vi "Argos_K_0v8.vi"(0 "PID 1 COM":refnum<visa-resource-name>="COM1", 1 "Setpoint\n START":bool, 2 "Write to File":bool, 3 "SP 1 input (°C)":dbl=20.0 min=0.0 max=1300.0, 4 "Intervall (s)":u32=1 max=600, 5 "Write/\nRead":bool=TRUE, 6 "Delay (ms)":u32=500 min=100 max=600000, 7 "Auto Tune":bool, 9 "Standby":bool, 11 "Reset\nSTOP":bool, 12 "ON":bool=TRUE caption="OFF", 13 "Get Values":bool, 15 "File Path":path) -> (8 "(°C)":dbl format="%#.3f", 14 "SP 1 is (°C)":dbl)   [LabVIEW 2013]
doc: "1. Verwendung\n\nDas Programm dient der Steuerung und Abfrage des Thermocontrollers I3252 und dem Auslesen von zwei VC 840 Messgeräten und einem Druckmessgerät Pfeiffer Single Gauge. \nDie Messgeräte werden Standardmäßig ausgelesen und erst nach Betätigung des Schalters \"Write to File\" in einer Textdatei abgespeichert. Das Eingabefeld \"Intervall\" legt den Abstand der Messpunkte fest.\nDer Setpoint für den Thermocontroller wird erst nach Betätigung des Tasters \"Setpoint START\" übernommen und angesteuert. Er wird ind den EEPROM des Gerätes geschrieben. Die Regelung kann mit Hilfe des Schalters \"Standby\" unterbrochen werden. Durch den Taster \"Reset STOPP\" kann der Setpoint aus dem EEPROM gelöscht werden.\nDie Eingabeflächen \"Constant\" und \"Thickness\" dienen der Berechnung des spezifischen Widerstands.\nDie Eingabeflächen \"User\" und \"Sample\" werden in den Header der Textdatei übernommen.\nDer Indikator \"File Path\" zeigt den aktuellen Speicherort der Textdatei an. Dieser wird nach ausschalten des Schalters \"Write to File\" gelöscht. Bei erneuten Schreiben muss ein neuer Speicherort gewählt werden. Bei Wahl desselben Speicherorts werden sämtliche bereits gespeicherte Daten gelöscht.\n\n\n2. Erläuterungen zum Blockdiagramm\n2.1 äußere Sequenz\nDie äußerte Sequenz besteht aus fünf Frames. Der erste dient der Initialisierung der Ports. Der zweite dient als Verzögerung um dem Programm genug Zeit zu geben die Ports zu öffnen. Jedoch senden die beiden VC 840 bereits Informationen an den Computer die in einem Puffer zwischengespeichert werden. Im dritten Frame wird dieser Puffer geleert. Somit kommt es zu keinem Framing Error. Desweiteren wird in diesem Frame die Startzeit der Messungen genommen. Im vierten Frame wird die eigentliche Messung und Verarbeitung der Daten durchgeführt. Die while-Schleife wird nur durch Auftreten eines Fehlers oder durch Betätigung des Stopbuttons auf dem Front Panel in der oberen linken Ecke unterbrochen. Im fünften und letzten Frame werden die Ports wieder geschlossen und beim Auftreten eines Fehlers wird das Programm automatisch gestoppt. Falls kein Fehler auftritt wird die Sequenz von vorne abgearbeitet.\n\n2.2 while-Schleife und innere Sequenz\n2.2.1 \"Event Structure\"\n2.2.1.1 Allgemein\nDer erste Frame beinhaltet ein \"Event Structure\". Dieser reagiert auf insgesamt elf verschiedene Ereignisse. Falls keines dieser Ereignisse auftreten sollte, warte die Struktur eine Millisekunde bevor die \"Event Structure\" verlassen wird. Die übrigen Ereignisse treten ein, wenn der entsprechende Kontroller eine Werteänderung erfährt.\n\n2.2.1.2 Event: Setpoint\nDieser Case besteht von außen nach innen aus einer Stacked Sequence, einer for-Loop und einer Flat Sequence die wiederum zwei \"Case Structures\" enthält. Als erstes wird bei dem Schalter \"Setpoint START\" der Blinkmodus aktiviert und bei dem Schalter \"Read Temperature\" deaktiviert. Danach folgt das eigentliche setzen des Temperatursollwerts. In der ersten Iteration wird dem Controller I3252 ein Schreibbefehl gesendet. Theoretisch kann der Setpoint in den RAM oder in den EEPROM geschrieben werden. Diese Auswahl erfolgt mit Hilfe des Schalters \"RAM\". Da das Schreiben in den RAM -Speicher aber aus diversen Gründen nicht erwünscht ist, wurde es nicht implementiert. Eine nachträgliche Implementierung ist aber leicht möglich, in dem die untere String-Konstante \"*P012\" durch \"*W012\" ersetzt wird. An diesem Befehl wird eine fünfstellige Hexadezimalzahl angehängt, die den Sollwert wiedergibt. Der Sollwert wird vorher mit zehn multipliziert, da das Komma standardmäßig nach der ersten Ziffer festgesetzt wurde (Bsp.: 800 wird gesendet um 80 einzustellen). Dieser Befehlsstrang wird an das Gerät mittels des SubVIs \"Comm_Interface\", auf welches später noch näher eingegangen wird, weitergegeben. Der durch das Gerät zurückgegebene String wird nicht verarbeitet.\nDie zweite Iteration dient dem Auslesen des eingestellten Sollwertes. Wahlweise kann der RAM- oder der EEPROM-Speicher ausgelesen werden. Die eigentliche Verarbeitung des Ausgabestrings erfolgt durch das SubVI \"Edit Setpoint\".\nDie Implementierung zur Einstellung des zweiten Setpoints erfolgt durch kopieren der ersten beiden Fälle und ersetzen der \"1\" im Befehf durch eine \"2\" (Bsp.: \"*P012\" zu \"*P022\"). Es darf aber nicht vergessen werden, dass dann ebenfalls die Anzahl der Iterationen angepasst werden muss.\nAls letztes wird der Blinkmodus des Schalters \"Setpoint START\" wieder deaktiviert.\n\n2.2.1.3 Event: Standby\nDieses Ereignis aktiviert bzw. deaktiviert als erstes den Blinckmodus des entsprechenden Schalters und sendet danach den Befehl zum aktivieren (\"*D03\") oder zum deaktivieren (\"*E03\") des Standbymodus an den Thermocontroller.\n\n2.2.1.4 Event: Set Command \nDer in das Feld \"Command shall be\" eingegebene Befehl wird an den Thermocontroller übermittlet. Die korrekte Form des Befehls ist im \"Communication Manuel\" nachzuschlagen. Das \"*\"-Zeichen wurde allerdings schon implementiert und muss somit nicht mit eingegeben werden.\n\n2.2.1.5 Event: Reset\nIn der ersten Iteration wird der Reset-Befehl an den Thermocontroller gesendet. In Folge wird der gesamte EEPROM-Speicher gelöscht. Deshalb wird in der zweiten Iteration der Setpoint aktualisiert. Dieser Befehl hat keinen Einfluss auf den RAM-Speicher. Die anschließende Wartezeit ist auf vier Sekunden festgesetzt und wurde empirisch ermittelt. Diese Zeit benötigt das Gerät um den Reset durchzuführen und für die Kommunikation wieder zur Verfügung zu stehen.\n\n2.2.1.6 Event: Auto Tune\nEs ist festgeschrieben, dass der Setpoint für die \"Auto Tune\"-Funktion wenigstens 20°C über der aktuellen Temperatur liegt. Deshalb wird zunächst der aktuelle Temperaturwert ausgelesen. Im zweiten Schritt werden zu diesem Wert zwanzig addiert und der Setpoint wird in den RAM-Speicher geschrieben. Das Schreiben in diesen Speicher ist nötig, da die \"Auto Tune\"-Funktion\" erst nach einem Reset startet. Im dritten Schritt wird der eigentliche Befehl für den \"Auto Tune\" gesendet (siehe dazu \"Communication Manuel\" S.27). Als vierte und letzte Iteration der for-Schleife folgt der bereits erwähnte Reset-Befehl. Der Temperatursollwert, der im RAM-Speicher eingetragen ist, muss zum Schluss wieder auf 0°C gesetzt werden. Die Zeit für die Ausführung des \"Auto Tune\"-Befehls wurde empirisch ermittelt und 45 s festgesetzt.\n\n2.2.1.7 Event: Write LOW/HI\nDieses Ereignis setzt die am Analogausgang anliegende Spannung fest. Normalerweise beträgt dieser Spannungswert 0-10 V. Das angeschlossene Netzteil verträgt aber maximal nur 2,3 V. Aus diesem Grund wird der \"%HIGH\" auf 23 gesetzt. Somit beträgt die maximal anliegende Spannung nur noch 23% von der maximal möglichen, d.h 2,3V. Ein niedrigerer Wert ist jederzeit möglich, genauso wie ein höherer für den Parameter \"%LOW\". Diese werden zunächst nacheinander in den RAM-Speicher geschrieben und anschließend wieder ausgelesen.\n\n2.2.1.8 Event: Set PID\nDie Werte für den PID-Regler können sowohl mit Hilfe der \"Auto Tune\"-Funktion, als auch manuell eingestellt werden. Es wird wiederum zwischen dem Schreiben in den RAM- und dem EEPROM-Speicher unterschieden. Zunächst werden die Werte für \"P\", \"I\" und \"D\", in dieser Reihenfolge, gesetzt und danach die aktuellen Werte ausgelesen.\n\n2.2.1.9 Event: Get Values\nDieses Ereignis hat zur Folge, dass die Werte für \"P\", \"I\", \"D\", \"%LOW\", \"%HIGH\" und des Setpoints wahlweise aus dem RAM- oder EEPROM-Speicher gelesen werden. Die aktuellen Werte werden nicht nur in die entsprechenden Anzeigefelder übernommen, sondern auch in die entsprechenden Eingabefelder, mit Ausnahme des Temperatursollwerts. \n\n2.2.1.10 Event: RAM\nPrinzipiell kann zwischen dem Schreiben in den RAM- oder EEPROM-Speicher des Thermocontrollers gewählt werden. Die entsprechende Schalterposition auf dem Frontpanel zeigt den aktuell verwendeten Speicher an. Die Anzeigewerte werden bei jedem Umschalten aktualisiert und sind im entsprechenden Speicher eingetragen. Die Implementierung ist identisch mit der des Ereignisses \"Get Values\". Es gilt zu beachten, dass die Werte für \"%LOW\" und \"%HIGH\" nur in den RAM-Speicher geschrieben werden können und somit auch nur aus diesem ausgelesen werden können.\n\n2.2.1.11 Event: Set Gauge to Zero\nMit Hilfe der SubVIs \"Get Pressure\" und \"Offset Display\" werden die Werte für den alten und den neuen Offset und der durch den zweiten Drucksensor ermittelt Druck ermittelt. \n\n2.2.1.12 Event: Write to File\nSollte der Schalter \"Write to File\" aktiviert werden, d.h. Schalterposition oben, so wird zunächst durch das SubVI \"Header\" ein Header für die unter \"File Path\" definierte Datei angelegt. Alle Werte, die bereits in der entsprechenden Datei stehen, werden dabei gelöscht.\n\n2.2.2 \"Timed Structures\"\nIm dritten Frame der inneren Sequenz werden die Werte für Zeitpunkt, Temperatur, Spannung, Strom und Druck ermittelt. Damit die Werte zum gleichen Zeitpunkt aufgenommen werden, werden \"Timed Sequences\" eingesetzt. Mit dem entsprechenden Schalter auf dem Front Panel unter dem Tab \"Settings\" kann gewählt werden, ob das entsprechende Gerät ausgelesen werden soll oder nicht. Die einzelnen Sequenzen werden parallel abgearbeitet, womit die Prozesszeit von diesem Frame durch der zeitintensivsten Sequenz abhängt. Dies ist in aller Regel das Auslesen der Temperatur, da ein \"Delay\" von 500 ms oder größer benötigt wird, um den Controller ordentlich ansprechen zu können.\nDie Systemzeit wird durch das SubVI \"System Time in Seconds\" in Sekunden umgerechnet und der in dem Parameter \"Starttime\" gespeicherte Wert wird abgezogen. Somit werden die Sekunden seit dem Start des Programms gezählt.\n\n2.2.3 restlichen Frames\nIm zweiten Frame wird das Intervall zwischen den einzelnen Messwerten festgelegt. Dabei wird der Wert des Parameters \"Delay\" abgezogen. Dieser Wert beträgt im Normalfall 500 ms und ist somit nicht vernachlääsigbar.\nDer Vierte Frame beinhaltet die Umrechnung des Temperatur-Strings in einen Temperaturwert durch das SubVI \"Edit Tmperature\", die Berechnung des spezifischen Widerstands durch das SubVI \"Resistivity Calculation\" und die Überprüfung des Druckwerts. Auch werden die neu gewonnen Werte in das entsprechende Shift-Register übernommen. Falls der Druckwert einen in dem Parameter \"Pressure Limit (mbar)\" festgelegten Grenzwert überschreiten sollte, wird der Thermocontroller automatisch in den Standby-Modus versetzt. Des Weiteren wird der Schalter \"Standby\" solange gesperrt, wie der Druck oberhalb des Grenzwertes liegt. Wenn der Druck wieder unter den Grenzwert gesunken ist, wird der Standby-Befehl nicht automatisch aufgehoben, sondern muss vom Benutzer durch Betätigung des entsprechenden Schalters gegeben werden.\nIm fünften Frame werden die Diagramme erstellt. Dabei wird jedes Mal von neuem das gesamte Shift-Register als Graph dargestellt. Weiterhin werden die Messwerte in ein 1D-Array geschrieben.\nDer sechste und letzte Frame beinhaltet den eigentlich Schreibvorgang der Messwerte in eine Textdatei und die Überprüfung ob ein Fehler vorliegt.\n\n2.3 SubVIs\n2.3.1 Allgemein\nDie SubVIs für die Messgeräte VC840 und das Druckmessgerät wurden aus anderen Quellen übernommen. \n\n2.3.2 \"Header\"\nIn den Header wird zunächst das aktuelle Datum und die aktuelle Zeit übernommen. Die ausgewählte Datei wird dabei überschrieben. Danach wird der Name des Benutzers und der Probe übernommen. Zum Schluss werden die Einheiten in einer Reihe, durch einen Tabulator getrennt, in den Header geschrieben.\n\n2.3.3 \"I3252 Comm Interface\"\nDieses VI stellt die Kommunikation mit dem Thermocontroller her und gibt den Ausgabe-String zurück.\n\n2.3.4 \"I3252 Edit Setpoint\"\nIm Ausgabe-String vom Thermocontroller ist an der vierten Stelle die Stelle des Dezimalpunktes verschlüsselt. Dieses Hexadezimalzahl wird herausgefiltert und an ein \"ENUM Controller\" übergeben. Dieser weist der Hexadezimalzahl eine Nummer zu, mit welcher ein Wert aus einem Array entnommen wird. Dieser Wert dient als Quotient. Der tatsächliche Wert kann somit errechnet werden.\n\n2.3.5 \"I3252 Edit Temperature\"\nDer Temperatur-String, der vom Thermocontroller zurückgegeben wird, wird in eine Dezimalzahl umgewandelt. Manchmal kommt es aus zu Dropouts, die durch dieses Programm herausgefiltert werden. Der letzte Wert wird dabei in einer \"Feedback Node\" gehalten unter der Annahme, dass sich der Temperaturwert nicht sprunghaft ändert.\n\n2.3.6 \"Resistivity Calculation\"\nDer spezifische Widerstand wird nach folgender Formel ausgerechnet. Dabei entspricht t der Dicke der Probe und C ist eine Konstante.\nrho=C*pi*t*U/(ln( 2)*I)\n\n2.3.7 \"System Time in Seconds\"\nZunächst wird die aktuelle Systemzeit ausgelesen. Danach wird diese in Stunden, Minuten und Sekunden aufgeteilt, alles in Sekunden umgerechnet und letztendlich addiert."
uses:
  <vilib>/Platform/TimedLoop/XDataNode/timing_clust.ctl
  <vilib>/Platform/TimedLoop/XDataNode/nitl_modes.ctl
  <vilib>/Platform/TimedLoop/XDataNode/wakeup.ctl
  <vilib>/Instr/_visa.llb/VISA Configure Serial Port (Instr).vi
  <vilib>/Platform/TimedLoop/scheduler/LVUserAPI/_suppVIs/Create_1kHz_TSource.vi
  <vilib>/Utility/file.llb/Write To Spreadsheet File (DBL).vi
  <vilib>/Platform/TimedLoop/XDataNode/XDataNode.xnode
  <vilib>/Platform/TimedLoop/XDataNode/XDNodeRunTimeDep.lvlib
  Argos0v7/Dependencies/Pfeiffer TPG261+262 Single+Dual Gauge/Dual Gauge.lvlib
panel:
  out "Thermocouple (Sample holder 1) 2":cluster{dbl[], dbl[]}(graph)
  out "(°C) 2":dbl format="%#.3f"
  out "appended array":dbl[](array[numeric])
  in  "Tab Control":T1(tab)
  out "SP 2 is (°C)":dbl
  in  "SP 2 input (°C)":dbl=20.0 min=0.0 max=1300.0
  in  "Standby\n2":bool
  in  "Setpoint\n START\n2":bool
  out "Pirani (VVP1 Scroll)":cluster{dbl[], dbl[]}(graph)
  in  "Thickness (nm)":dbl min=0.0
  in  "4PP constant":dbl min=0.0 max=5.0
  in  "Sample":string
  in  "User":string
  out "Thermocouple (Sample holder 1)":cluster{dbl[], dbl[]}(graph)
  out "current time (s)":dbl
  out "data logger intervall (s)":dbl
  out "loop time (s)":dbl
  in  "stop":bool
  out "CMR275 Baratron":cluster{dbl[], dbl[]}(graph)
  out "Pressure Baratron 2":dbl format="%#_4e"
  out "PKR251 FullRange":cluster{dbl[], dbl[]}(graph)
  out "Pressure FullRange 2":dbl format="%#_3e"
  out "Pressure Pirani 2":dbl format="%#_3e"
  in  "Reset\nSTOP 2":bool
  out "Pressure OpenPort":cluster{dbl[], dbl[]}(graph)
  out "Pressure OpenPort2":dbl caption="current"
  out "% HIGH Istwert 2":u32
  out "% LOW Istwert 2":u32
  in  "% High Sollwert 2":u32=23 max=24
  in  "% LOW Sollwert 2":u32 max=25
  in  "RAM 2":bool=TRUE caption="EEPROM"
  out "D (Rate) IstWert 2":u32
  out "I ( Reset1) Istwert 2":u32
  out "P (PB1) Istwert 2":u32 caption="actual value"
  in  "D (Rate) Sollwert 2":u32 max=3999
  in  "I ( Reset1) Sollwert 2":u32 max=3999
  in  "P (PB1) Sollwert 2":u32 caption="set value" max=9999
  in  "ON 2":bool=TRUE caption="OFF"
  in  "PID 2 COM":refnum<visa-resource-name>="COM1"
  in  "Baud Rate 2":u32=9600
  in  "Data Bits 2":u16=7 min=5 max=8 step=1
  in  "Parity 2":u16(ring)=1 items=["None", "Odd", "Even", "Mark", "Space"]
  in  "Stop Bits 2":u16(ring)=10 items=["1.0"=10, "1.5"=15, "2.0"=20]
  in  "Flow Control 2":u16(ring) items=["None"=0, "XON/XOFF"=1, "RTS/CTS"=2, "DTR/DSR"=4]
  in  "Delay (ms) 2":u32=500 min=100 max=600000
  in  "Write/\nRead \n\n2":bool=TRUE
  out "status 2":bool caption="Status"
  out "code 2":i32 caption="Code"
  out "code":i32 caption="Code"
  out "status":bool caption="Status"
  in  "Set Gauge to Zero":bool
  out "Status Gauge 1#2":i32(ring) items=["data OK", "underrange", "overrange", "sensor error", "sensor off", "no sensor", "ID error"]
  out "Pressure Gauge 1#2":dbl format="%.3e"
  out "Pressure Gauge 1#1":dbl format="%.3e"
  out "Status Gauge 1#1":i32(ring) items=["data OK", "underrange", "overrange", "sensor error", "sensor off", "no sensor", "ID error"]
  in  "TPG 1 COM":refnum<visa-resource-name>="COM5"
  in  "Pressure Limit (mbar)":dbl=1.0 min=0.0 max=1100.0
  out "Current Offset (mbar)":dbl
  in  "ON (TPG 2)":bool=TRUE caption="OFF"
  in  "ON (TPG 1)":bool=TRUE caption="OFF"
  in  "ON":bool caption="OFF"
  in  "VC 840 2":refnum<visa-resource-name>="COM7"
  out "Reading 2":dbl format="%_4f"
  out "Mode 2":enum16{"?", "Diode", "Beep", "DC", "AC"}(ring)
  out "Unit 2":string
  in  "VC 840 1":refnum<visa-resource-name>="COM7"
  out "Reading 1":dbl format="%_4f"
  out "Mode 1":enum16{"?", "Diode", "Beep", "DC", "AC"}(ring)
  out "Unit 1":string
  out "Status 1":T2
  out "Status 2":T2
  in  "ON":bool caption="OFF"
  out "% HIGH Istwert":u32
  out "% LOW Istwert":u32
  in  "% High Sollwert":u32=23 max=24
  in  "% LOW Sollwert":u32 max=25
  in  "RAM":bool=TRUE caption="EEPROM"
  out "D (Rate) IstWert":u32
  out "I ( Reset1) Istwert":u32
  out "P (PB1) Istwert":u32 caption="actual value"
  in  "D (Rate) Sollwert":u32 max=3999
  in  "I ( Reset1) Sollwert":u32 max=3999
  in  "P (PB1) Sollwert":u32 caption="set value" max=9999
  in  "Set Command":bool
  in  "Set PID":bool
  in  "Write LOW/HI":bool
  in  "Flow Control":u16(ring) items=["None"=0, "XON/XOFF"=1, "RTS/CTS"=2, "DTR/DSR"=4]
  in  "Stop Bits":u16(ring)=10 items=["1.0"=10, "1.5"=15, "2.0"=20]
  in  "Parity":u16(ring)=1 items=["None", "Odd", "Even", "Mark", "Space"]
  in  "Data Bits":u16=7 min=5 max=8 step=1
  in  "Baud Rate":u32=9600
  out "Command output":string
  in  "Command input":string
  in  "TPG 2 COM":refnum<visa-resource-name>="COM6"
  out "Pressure Gauge 2#2":dbl format="%.3e"
  out "Pressure Gauge 2#1":dbl format="%.3e"
  out "Status Gauge 2#2":i32(ring) items=["data OK", "underrange", "overrange", "sensor error", "sensor off", "no sensor", "ID error"]
  out "Status Gauge 2#1":i32(ring) items=["data OK", "underrange", "overrange", "sensor error", "sensor off", "no sensor", "ID error"]
  out "Command output 2":string
  in  "Command input 2":string
  in  "Set Command\n\n 2":bool
  in  "Auto Tune 2":bool
  in  "Set PID 2":bool
  in  "Write LOW/HI 2":bool
  in  "Get Values 2":bool
  out "Current":cluster{dbl[], dbl[]}(graph)
  out "Voltage":cluster{dbl[], dbl[]}(graph)
  out "Voltage (V)":dbl format="%.4e"
  out "Current (A)":dbl format="%.4e"
  out "Resistivity":cluster{dbl[], dbl[]}(graph)
  out "Resistivity (Ohm*cm)":dbl format="%.3e"
  # "PID 1"
  # "set \nvalue"
  # "actual \nvalue"
  # "T (°C)"
  # "PID 2"
  # "mbar"
  # "Set \nValue\n2"
  # "Actual \nvalue 2"
  # "T (°C)"
  # "mbar"
  # "mbar"
  # "mbar"
  # "Pressure Measurement \n(Pfeiffer TPG261)"
  # "PID Controller (Omega Newport i3252)"
  # "PID Controller 2 (Omega Newport i3252)"
  # "limit (mbar)"
  # "P"
  # "I"
  # "D"
  # "% Low"
  # "% High"
  # "Multimeter\n#1 (VC 840)"
  # "Multimeter\n#2 (VC 840)"
  # "P"
  # "I"
  # "D"
  # "% Low"
  # "% High"
  # "Authors:  Daniel Schuster (sir-dan@web.de)\n                 Steffen Cornelius (s.cornelius@hzdr.de)\n                 Nico Spahn (x)\n\n                 premade SubVIs for readout of Pfeiffer gauge and VC840 Multimeters were used\n                 SubVI \"I3252_Comm_Interface\" is based on a modified Labview example\n\nRelease:  v1.0    \n\nVersion History:\n\nv1.1  -    28.06.2011\n             - Format des Files geändert von %.3f auf %g\n             - maximale Eingabewerte für PID begrenzt\nv1.2  -    12.07.2011\n             - Anzeige p,rho, U, V auf Scientific geändert\n             - y-Achse p,rho auf Log geändert\n             - numerische Zeitanzeige hinzugefügt\n             - 4PP Constant: pi/ln(2)=4,532 set as the default value\nv1.3  -    25.07.2011\n             - Zeitvariable auf EXT geändert, um Sprünge in Diagrammen loszuwerden\nv1.4  -   27.07.2011\n             - ALLE Variablen auf DBL zurückgesetzt wegen Formatierungsproblem im File\n             - Zeitberechnung neu gemacht (Tick count differenzen) -> Zeitsprünge korrigiert ?\n             - Delay/Intervall überarbeitet\nv1.5  -   05.12.2012\n                - Austausch der alten Pfeifer SubvIs durch neue -> nun alle 4 Kanäle des DualGauge\n                                                                                                         Controllers gleichzeitig auslesbar\n                - neue Pfeiffer SubVIs verwendet in Druckwertauslesung und Offset Berechnung des Baratron\n                  Druckes (COM5 Sensor1)\n                - Neuarragement des GUI -> FullRange und Baratron neben Temperatur auf Haupseite zu sehen\n                                                                   Pirani und OpenPort auf Meas.2 zu sehen\n                                                                   Diagnose Seite umfasst nun auch Widerstandsdiagramm\n                - Änderungen der Settingseite -> nun alle 4 Drucksensoren mit aktuellem Messwert und Gerätestatus\n                                                                           zu sehen\n                - The readout of the PID-Temperature Controller and the VC840 Multimeters was not modified\nv1.73  -  18.10.2013\n                - Layout Änderungen\nv.1.8   -  19.01.2014\n                - Änderung Layout Settings Tab\n                - Trennung der beiden TPG Dual Gauge Controls\n                -"
  # "Version 1.73    - last change 18.10.2013"
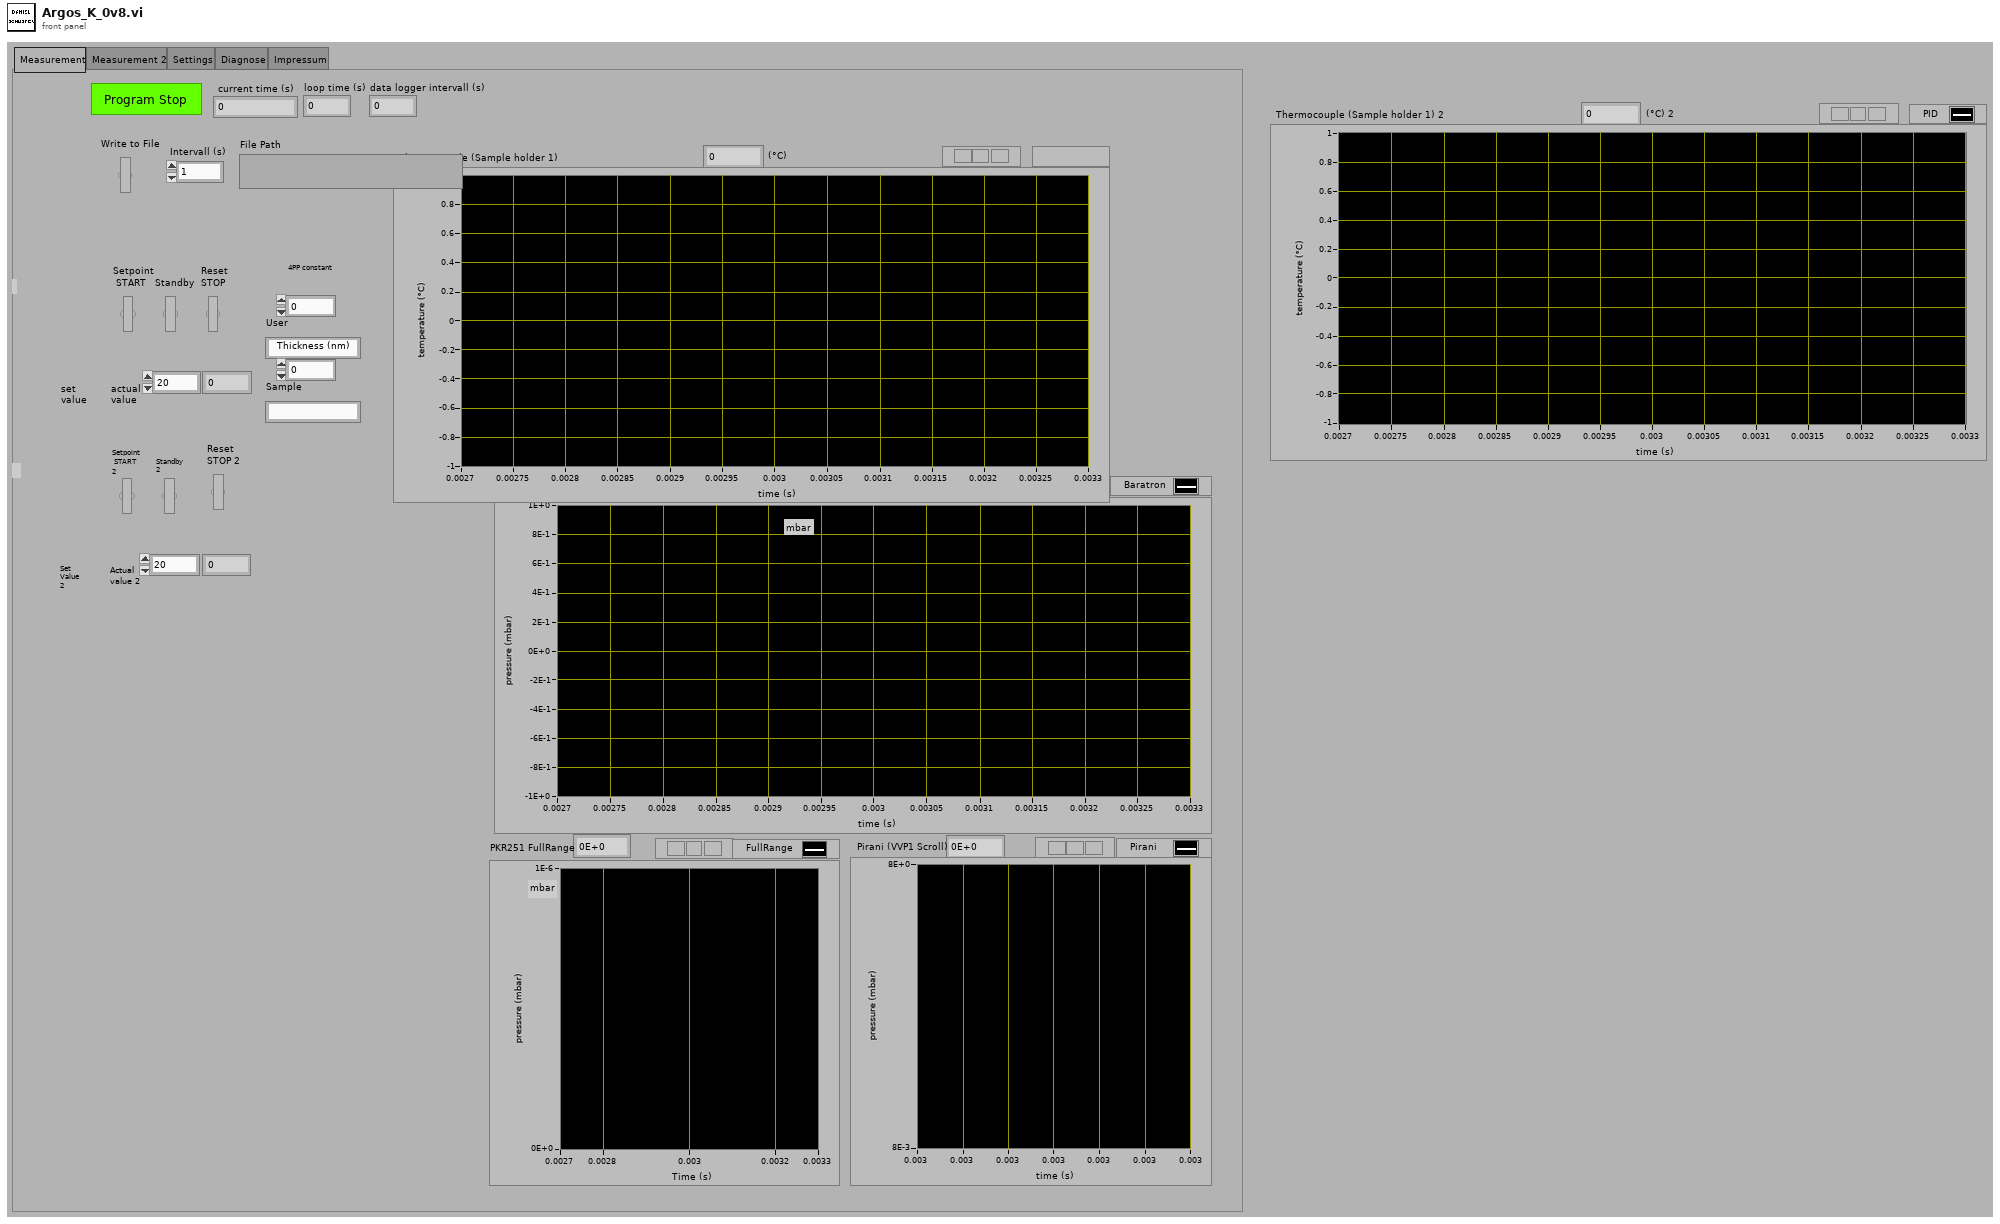
[diagram p1: front panel]
types:
  T1 = enum32{"Measurement", "Measurement 2", "Settings", "Diagnose", "Impressum"}
  T2 = cluster{"Low Bat":bool, "Auto":bool, "Delta":bool, "Hold":bool, "RS232":bool}
  T3 = typedef "XDNodeRunTimeDep.lvlib/timing_clust.ctl" = cluster{"Expected End [f-1]":u64, "Actual End [f-1]":u64, "Finished Late? [f-1]":bool, "Expected End [i-1]":u64, "Actual End [i-1]":u64, "Finished Late? [i-1]":bool, "Expected Start [i]":u64, "Actual Start [i]":u64, "Expected Start [f]":u64, "Actual Start [f]":u64, "Source Name":string, "Structure Name":string, "Period":i64, "Deadline":i64, "Offset":i64, "Start":i64, "Priority":i32, "Timeout":i32, "Mode":T4, "Wakeup Reason":T5, "Error":errorcluster, "Source Type":string, "Secondary Source Type":string, "Global End Time":u64, "Global Start Time":u64, "Frame Duration":u64, "Iteration Duration":u64, "Assigned CPU":i32, "I/O Scan Engine Mode":u32}
  T4 = typedef "XDNodeRunTimeDep.lvlib/nitl_modes.ctl" = enum32{"No Change", "Process missed periods, maintain original phase", "Discard missed periods, maintain original phase", "Process missed periods, ignore original phase", "Discard missed periods, ignore original phase"}
  T5 = typedef "XDNodeRunTimeDep.lvlib/wakeup.ctl" = enum32{"Normal", "Aborted", "Asynchronous wakeup", "Timing source error", "Timed loop error", "Timeout"}
  T6 = enum8{"Enabled", "Disabled", "Disabled and Grayed Out"}
  T7 = cluster{"VISA resource name out":refnum<visa-resource-name>, "error out":errorcluster, "Delay (ms)":u32, "Write/\nRead":bool}
  T8 = cluster{"VISA resource name out":refnum<visa-resource-name>, "error out":errorcluster, "Delay (ms) 2":u32, "Write/\nRead \n\n2":bool}
  T9 = cluster{"TPG 2 COM":refnum<visa-resource-name>, "error out":errorcluster}
  T10 = cluster{"COM out":refnum<visa-resource-name>, "Cluster (Ausgang)":errorcluster}
  T11 = cluster{"Pressure Gauge#1":dbl, "Pressure Gauge#2":dbl}
  T12 = cluster{"TPG 1 COM":refnum<visa-resource-name>, "error out":errorcluster}
  T13 = cluster{"COM out":refnum<visa-resource-name>, "error out":errorcluster, "COM out":refnum<visa-resource-name>, "error out":errorcluster}
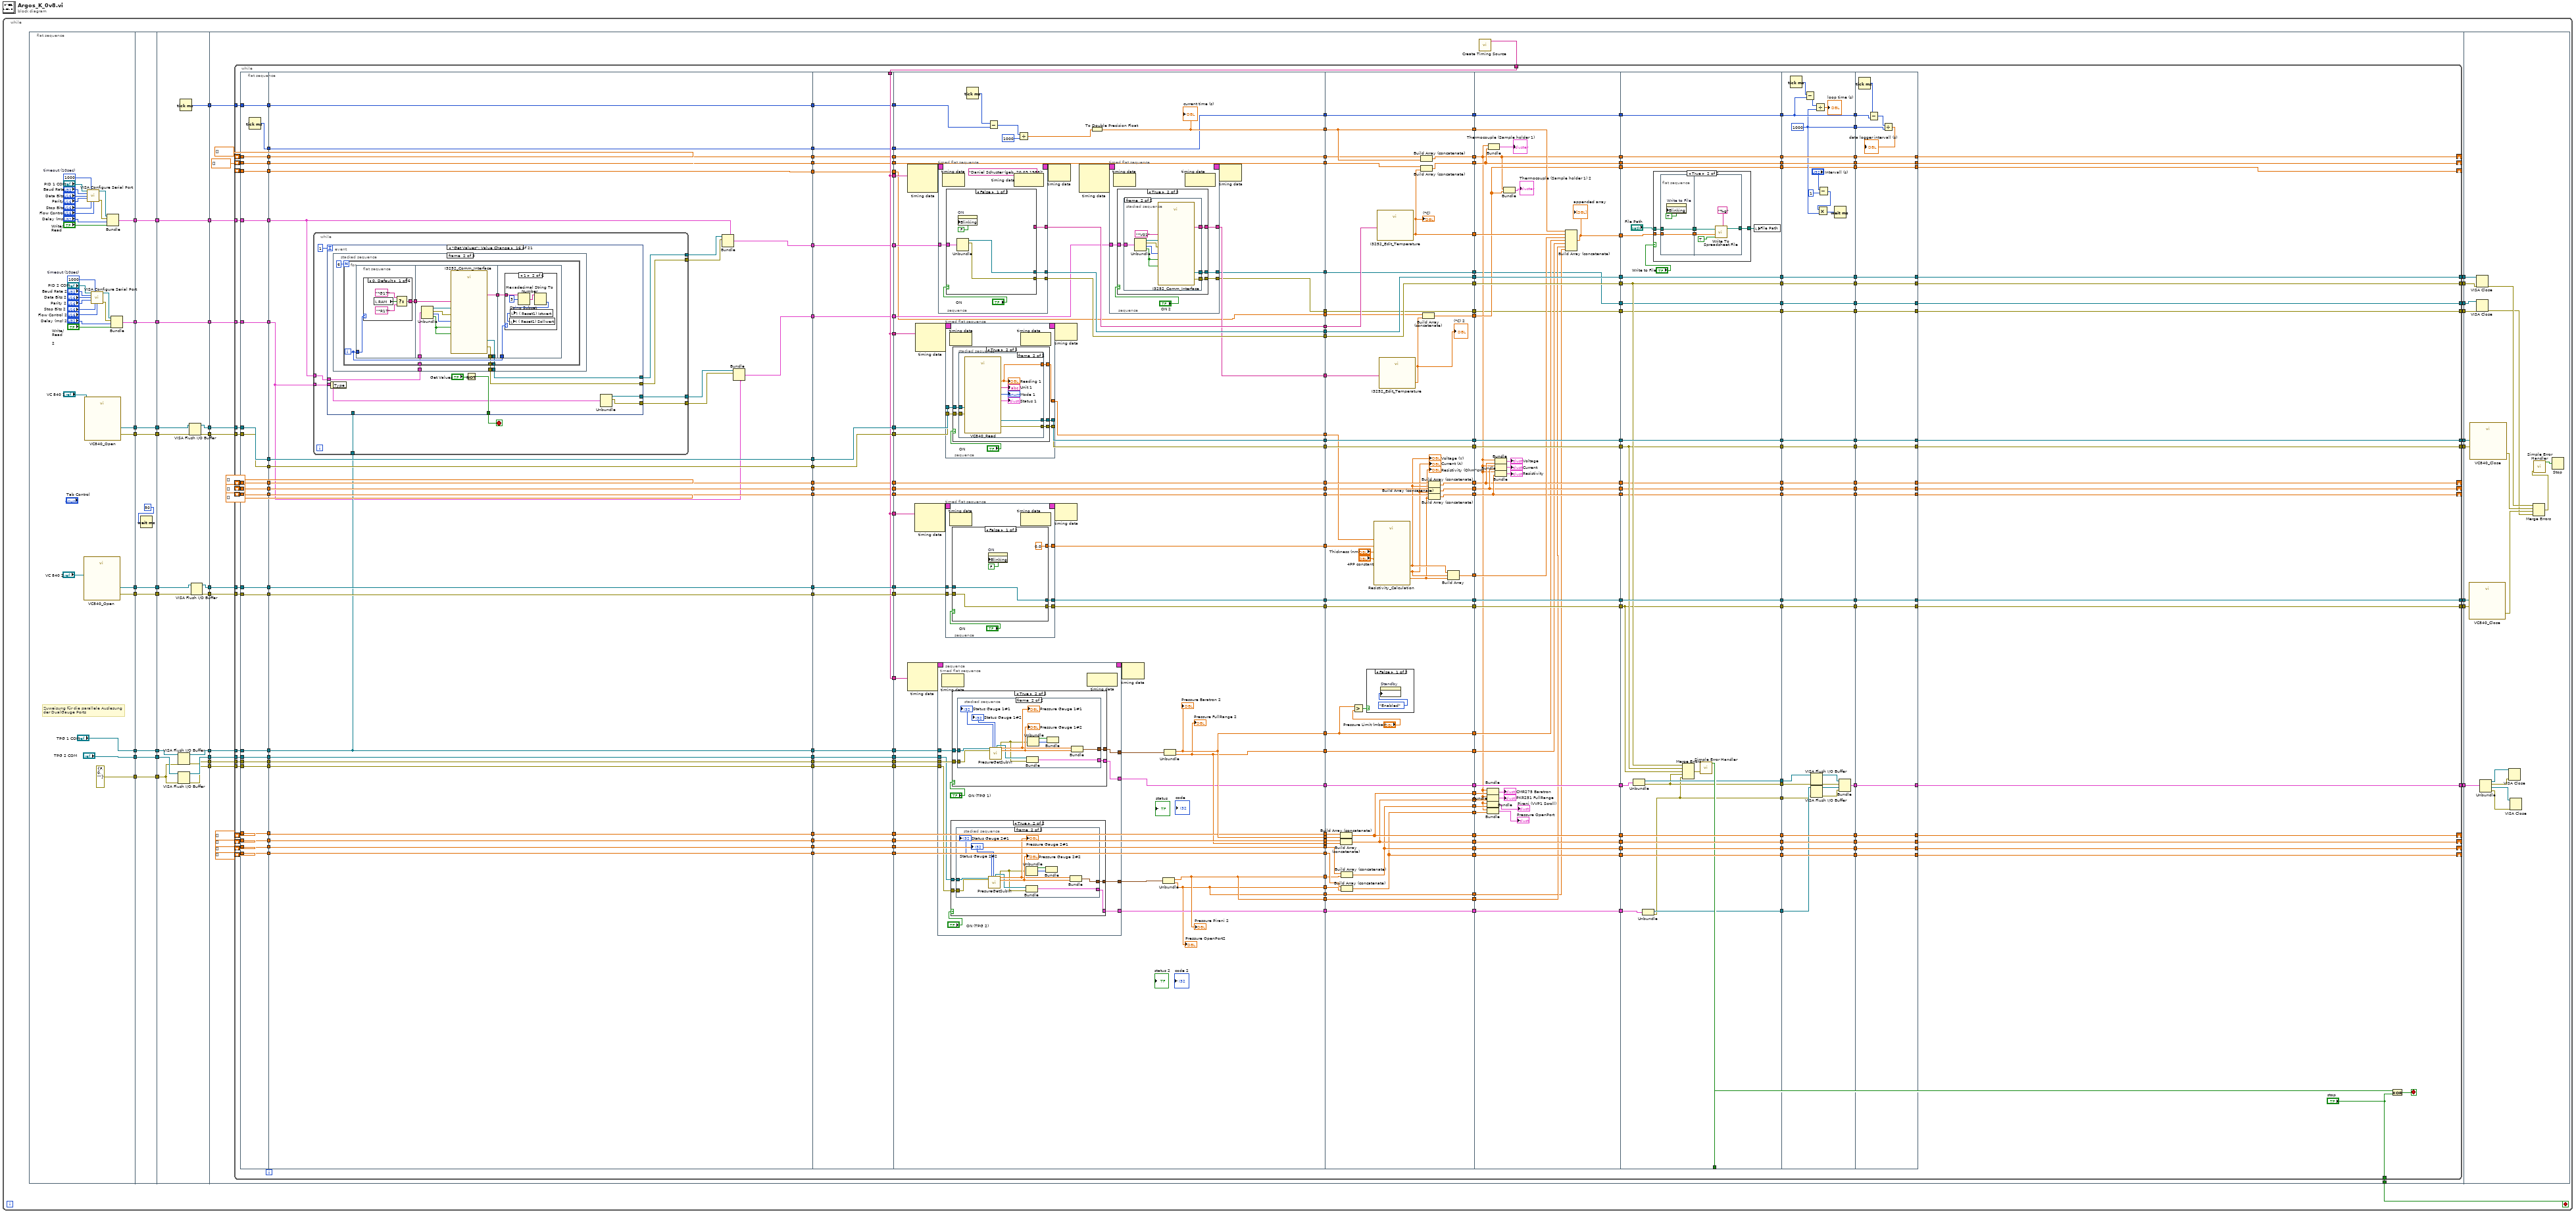
[diagram p0: block diagram]
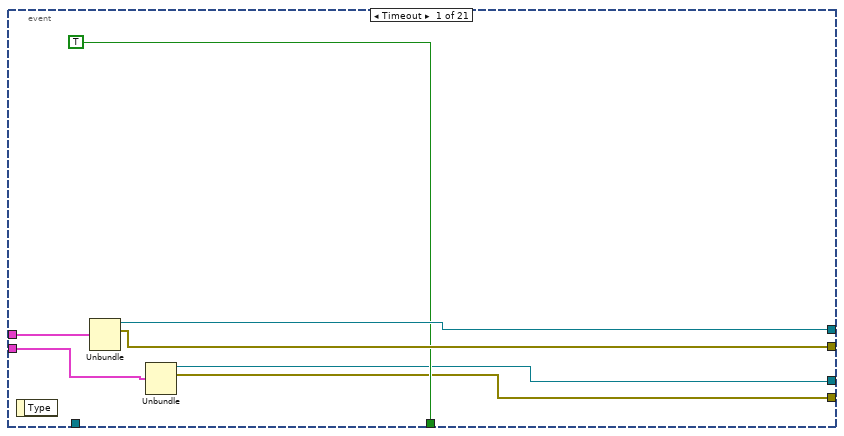
[diagram p2: hidden frame]
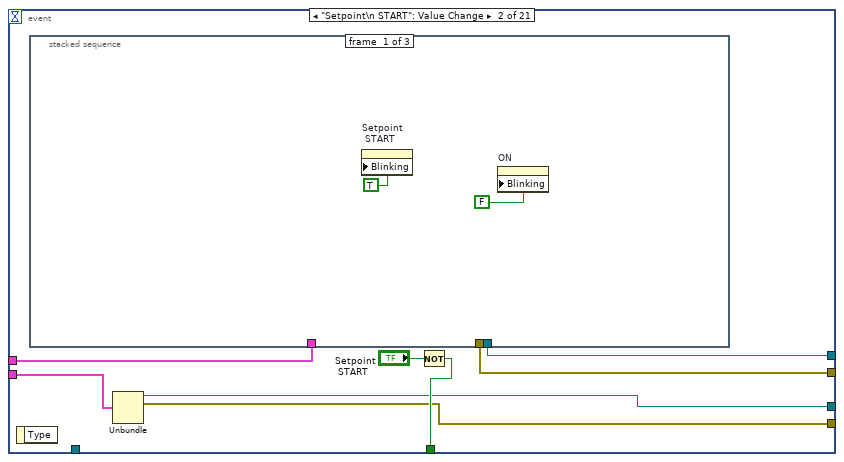
[diagram p3: hidden frame]
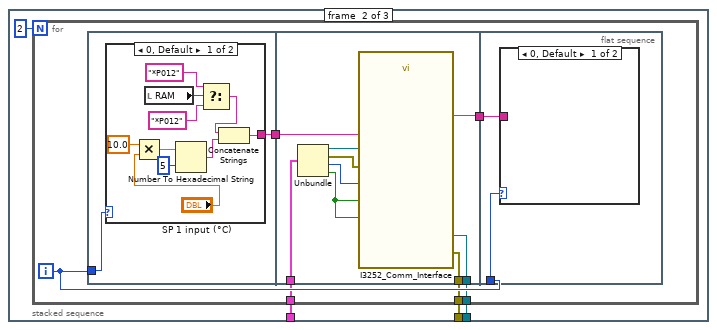
[diagram p4: hidden frame]
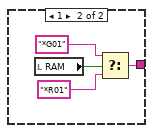
[diagram p5: hidden frame]
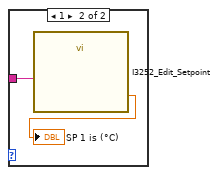
[diagram p6: hidden frame]
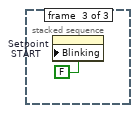
[diagram p7: hidden frame]
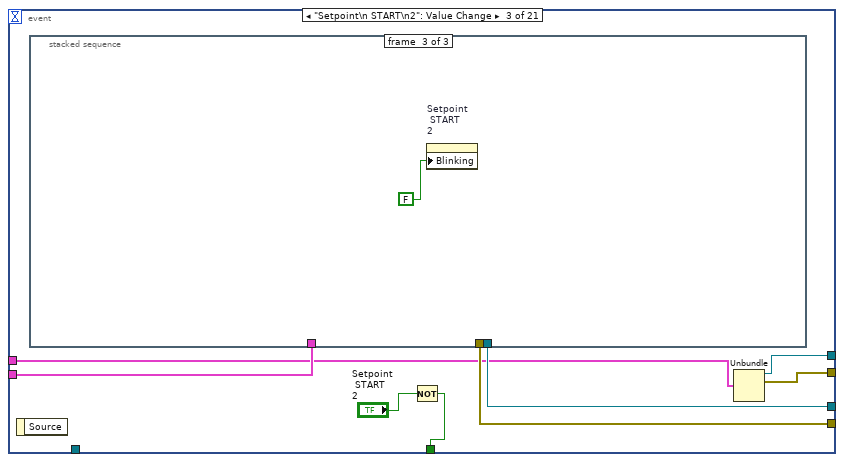
[diagram p8: hidden frame]
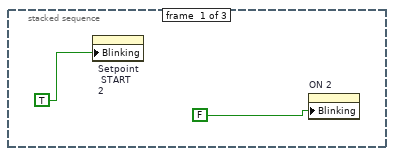
[diagram p9: hidden frame]
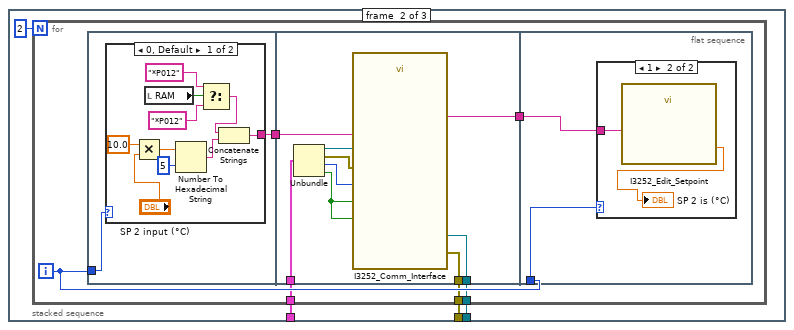
[diagram p10: hidden frame]
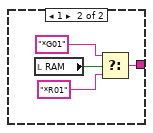
[diagram p11: hidden frame]
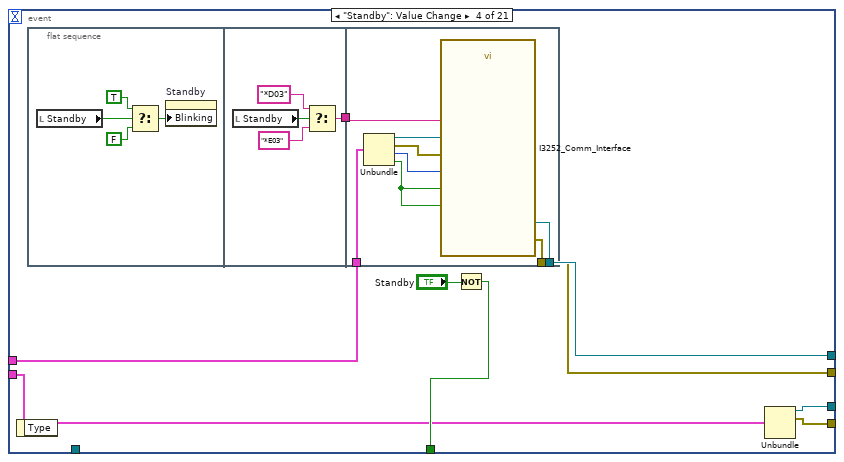
[diagram p13: hidden frame]
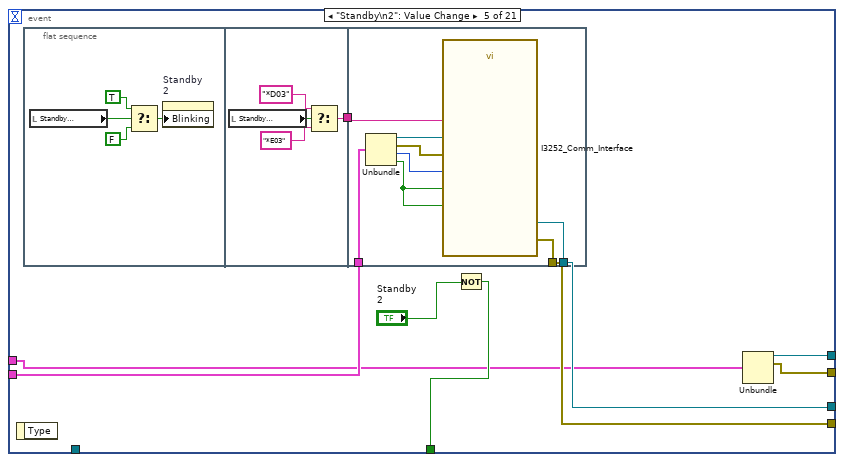
[diagram p14: hidden frame]
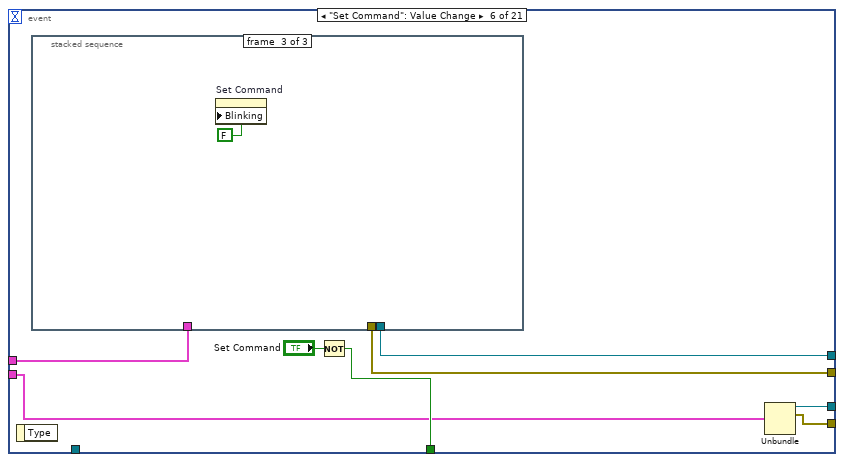
[diagram p15: hidden frame]
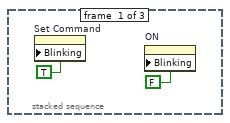
[diagram p16: hidden frame]
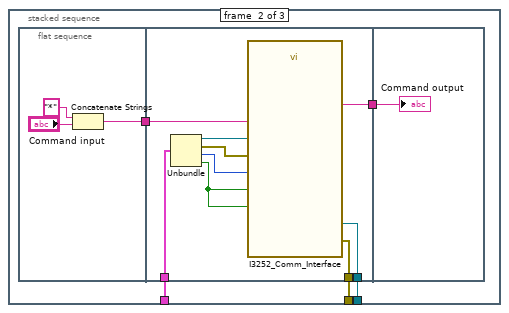
[diagram p17: hidden frame]
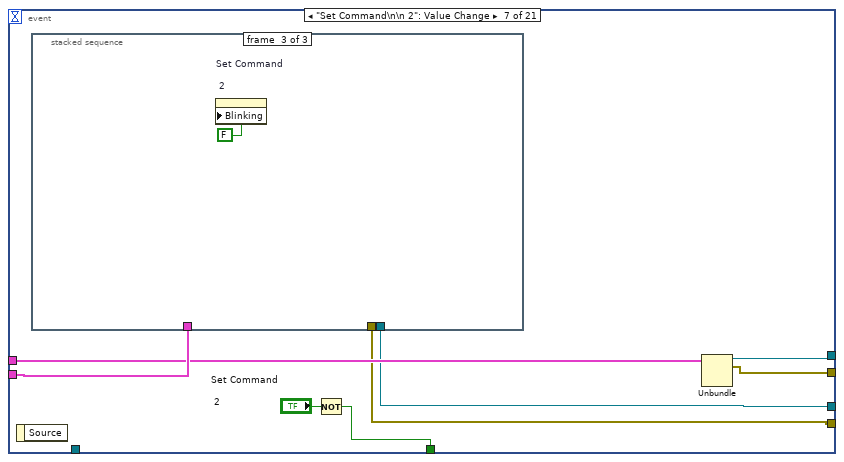
[diagram p18: hidden frame]
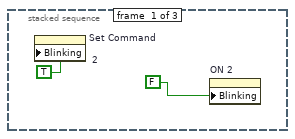
[diagram p19: hidden frame]
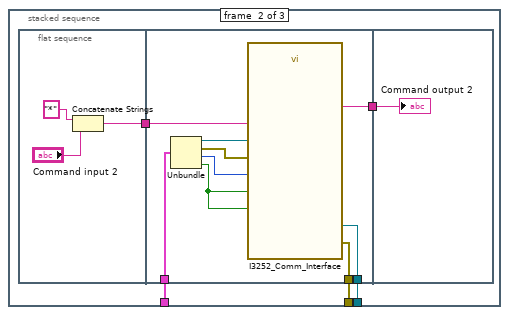
[diagram p20: hidden frame]
diagram:
  n1 = while {
    stop <- w11 stop-if-true
    n2 = flat-sequence {
      tunnel: [w71] -> w39
      tunnel: [w72] -> w38
      tunnel: [w57] -> w37
      tunnel: [w70] -> w36
      tunnel: [w69] -> w35
      tunnel: ["TPG 1 COM"] -> w34
      tunnel: ["TPG 2 COM"] -> w33
      tunnel: [errorcluster {"status"=FALSE, "code"=0, "source"=""} ("Fehler (Eingang)")] -> w8
      tunnel: [w40] -> w3
      tunnel: w39 -> [w82]
      tunnel: [w82] -> w32
      tunnel: w38 -> [w81]
      tunnel: [w81] -> w31
      tunnel: w37 -> [w80]
      tunnel: [w80] -> w30
      tunnel: w36 -> [w79]
      tunnel: [w79] -> w29
      tunnel: w35 -> [w78]
      tunnel: [w78] -> w28
      tunnel: [w76] -> w27
      tunnel: w34 -> [w76]
      tunnel: [w75] -> w26
      tunnel: w33 -> [w75]
      tunnel: [w74] -> w9
      tunnel: w8 -> [w74]
      tunnel: [w73] -> w4
      tunnel: w3 -> [w73]
      tunnel: w32 -> [w94]
      tunnel: [w93] -> w25
      tunnel: w31 -> [w95]
      tunnel: [w92] -> w24
      tunnel: w30 -> [w100]
      tunnel: [w100] -> w23
      tunnel: w29 -> [w97]
      tunnel: [w98] -> w22
      tunnel: w28 -> [w96]
      tunnel: [w99] -> w21
      tunnel: [w91] -> w20
      tunnel: [w89] -> w19
      tunnel: w27 -> [w90]
      tunnel: [w88] -> w18
      tunnel: w26 -> [w87]
      tunnel: w9 -> [w86]
      tunnel: [w85] -> w7
      tunnel: [w84] -> w6
      tunnel: [w83] -> w5
      tunnel: w4 -> [w83]
      tunnel: w25 -> [w131]
      tunnel: w24 -> [w130]
      tunnel: w23 -> [w129]
      tunnel: w22 -> [w127]
      tunnel: w21 -> [w126]
      tunnel: [w125] -> w17
      tunnel: [w124] -> w16
      tunnel: [w123] -> w15
      tunnel: [w122] -> w14
      tunnel: [w121] -> w13
      tunnel: [w120] -> w12
      tunnel: w20 -> [w114]
      tunnel: w19 -> [w113]
      tunnel: w18 -> [w112]
      tunnel: [w107] -> w11
      tunnel: [w106] -> w10
      tunnel: w7 -> [w105]
      tunnel: w6 -> [w104]
      tunnel: w5 -> [w103]
      tunnel: [w102] -> w2
      tunnel: [w101] -> w1
      tunnel: w17 -> [w1956]
      tunnel: w16 -> [w1955]
      tunnel: w15 -> [w1958]
      tunnel: w14 -> [w1957]
      tunnel: w13 -> [w1960]
      tunnel: w12 -> [w1959]
      tunnel: w10 -> [w1953]
      tunnel: w2 -> [w1948]
      tunnel: w1 -> [w1947]
      frame #0 {
        w41 = u32 1000  # timeout (10sec)
        w58 = u32 1000  # timeout (10sec)
        # "Zuweisung für die parallele Auslesung\nder DualGauge Ports"
        n3 = call "VC840_Open.vi"("VISA resource name"="VC 840 2") -> ("error out"=w69:errorcluster, "VISA resource name out"=w70:refnum<visa-resource-name>)  [unwired: 1 in, 8 out]
        n4 = call "VC840_Open.vi"("VISA resource name"="VC 840 1") -> ("error out"=w72:errorcluster, "VISA resource name out"=w71:refnum<visa-resource-name>)  [unwired: 1 in, 8 out]
        n5 = call-poly "VISA Configure Serial Port"("VISA resource name"="PID 1 COM", "timeout (10sec)"=w58, "baud rate (9600)"="Baud Rate", "data bits (8)"="Data Bits", "parity (0:none)"="Parity", "stop bits (10: 1 bit)"="Stop Bits", "flow control (0:none)"="Flow Control") -> ("VISA resource name out"=w67:refnum<visa-resource-name>, "error out"=w68:errorcluster)  [unwired: 2 in, 5 out]
        n6 = call-poly "VISA Configure Serial Port"("VISA resource name"="PID 2 COM", "timeout (10sec)"=w41, "baud rate (9600)"="Baud Rate 2", "data bits (8)"="Data Bits 2", "parity (0:none)"="Parity 2", "stop bits (10: 1 bit)"="Stop Bits 2", "flow control (0:none)"="Flow Control 2") -> ("VISA resource name out"=w50:refnum<visa-resource-name>, "error out"=w51:errorcluster)  [unwired: 2 in, 5 out]
        n7 = Bundle("VISA resource name out"=w67, "error out"=w68, "Delay (ms)"="Delay (ms)", "Write/\nRead"="Write/\nRead") -> (w57:T7)  [unwired: 1 in]
        n8 = Bundle("VISA resource name out"=w50, "error out"=w51, "Delay (ms) 2"="Delay (ms) 2", "Write/\nRead \n\n2"="Write/\nRead \n\n2") -> (w40:T8)  [unwired: 1 in]
      }
      frame #1 {
        n9 = Wait (ms)(milliseconds to wait=u32 50) -> ()  [unwired: 1 out]
      }
      frame #2 {
        n10 = VISA Flush I/O Buffer(VISA resource name=w90, error in (no error)=w86) -> (VISA resource name out=w89:refnum<visa-resource-name>, error out=w85:errorcluster)  [unwired: 1 in]
        n11 = VISA Flush I/O Buffer(VISA resource name=w87, error in (no error)=w86) -> (VISA resource name out=w88:refnum<visa-resource-name>, error out=w84:errorcluster)  [unwired: 1 in]
        n12 = Tick Count (ms)() -> (millisecond timer value=w91:u32)
        n13 = VISA Flush I/O Buffer(VISA resource name=w94, error in (no error)=w95) -> (VISA resource name out=w93:refnum<visa-resource-name>, error out=w92:errorcluster)  [unwired: 1 in]
        n14 = VISA Flush I/O Buffer(VISA resource name=w97, error in (no error)=w96) -> (VISA resource name out=w98:refnum<visa-resource-name>, error out=w99:errorcluster)  [unwired: 1 in]
      }
      frame #3 {
        n15 = call-poly <vilib>:"Create Timing Source.vi"() -> ("name (out)"=w128:string)  [unwired: 10 in, 1 out]
        n16 = while {
          tunnel: w131 -> [w377]
          tunnel: w130 -> [w376]
          tunnel: w129 -> [w375]
          tunnel: w128 -> [w368]
          tunnel: w127 -> [w361]
          tunnel: w126 -> [w360]
          tunnel: [w356] -> w125
          tunnel: [w355] -> w124
          tunnel: [w353] -> w123
          tunnel: [w351] -> w122
          tunnel: [w349] -> w121
          tunnel: [w347] -> w120
          shift-right: [w320] -> _
          shift-left: dbl[] [] -> [w325]
          shift-right: [w298] -> _
          shift-left: dbl[] [] -> [w333]
          shift-right: [w322] -> _
          shift-left: dbl[] [] -> [w329]
          shift-right: [w295] -> _
          shift-left: dbl[] [] -> [w332]
          shift-right: [w292] -> _
          shift-left: dbl[] [] -> [w331]
          tunnel: w114 -> [w286]
          tunnel: w113 -> [w242]
          tunnel: w112 -> [w238]
          shift-right: [w196] -> _
          shift-left: dbl[] [] -> [w226]
          shift-right: [w194] -> _
          shift-left: dbl[] [] -> [w224]
          shift-right: [w192] -> _
          shift-left: dbl[] [] -> [w222]
          shift-right: [w190] -> _
          shift-left: dbl[] [] -> [w220]
          tunnel: ["stop"] -> w107
          tunnel: [w184] -> w106
          tunnel: w105 -> [w179]
          tunnel: w104 -> [w177]
          tunnel: w103 -> [w157]
          shift-right: [w149] -> _
          shift-left: _ -> [w147]
          tunnel: [w138] -> w102
          tunnel: [w132] -> w101
          stop <- w183 stop-if-true
          n17 = flat-sequence {
            tunnel: w286 -> [w389]
            tunnel: w325 -> [w390]
            tunnel: w329 -> [w391]
            tunnel: w331 -> [w392]
            tunnel: w332 -> [w393]
            tunnel: w333 -> [w394]
            tunnel: w360 -> [w395]
            tunnel: w361 -> [w396]
            tunnel: w375 -> [w397]
            tunnel: w376 -> [w398]
            tunnel: w377 -> [w399]
            tunnel: [w399] -> w285
            tunnel: [w398] -> w284
            tunnel: [w397] -> w283
            tunnel: [w396] -> w282
            tunnel: [w395] -> w281
            tunnel: [w394] -> w280
            tunnel: [w393] -> w279
            tunnel: [w392] -> w278
            tunnel: [w391] -> w277
            tunnel: [w390] -> w276
            tunnel: [w389] -> w275
            tunnel: [w388] -> w257
            tunnel: [w387] -> w243
            tunnel: w242 -> [w387]
            tunnel: [w386] -> w239
            tunnel: w238 -> [w386]
            tunnel: [w385] -> w227
            tunnel: w226 -> [w385]
            tunnel: [w384] -> w225
            tunnel: w224 -> [w384]
            tunnel: [w383] -> w223
            tunnel: w222 -> [w383]
            tunnel: [w382] -> w221
            tunnel: w220 -> [w382]
            tunnel: [w381] -> w180
            tunnel: w179 -> [w381]
            tunnel: [w380] -> w178
            tunnel: w177 -> [w380]
            tunnel: [w379] -> w158
            tunnel: w157 -> [w379]
            tunnel: [w378] -> w148
            tunnel: w147 -> [w378]
            tunnel: [w427] -> w374
            tunnel: [w426] -> w372
            tunnel: [w422] -> w370
            tunnel: [w421] -> w365
            tunnel: [w420] -> w363
            tunnel: [w419] -> w330
            tunnel: [w418] -> w326
            tunnel: [w417] -> w306
            tunnel: [w416] -> w303
            tunnel: [w415] -> w301
            tunnel: [w414] -> w287
            tunnel: w285 -> [w427]
            tunnel: w284 -> [w426]
            tunnel: w283 -> [w425]
            tunnel: w282 -> [w421]
            tunnel: w281 -> [w420]
            tunnel: w280 -> [w417]
            tunnel: w279 -> [w416]
            tunnel: w278 -> [w415]
            tunnel: w277 -> [w419]
            tunnel: w276 -> [w418]
            tunnel: w275 -> [w414]
            tunnel: [w413] -> w258
            tunnel: w257 -> [w413]
            tunnel: w243 -> [w411]
            tunnel: [w411] -> w240
            tunnel: w239 -> [w412]
            tunnel: [w412] -> w236
            tunnel: w227 -> [w410]
            tunnel: w225 -> [w409]
            tunnel: w223 -> [w408]
            tunnel: w221 -> [w407]
            tunnel: [w410] -> w219
            tunnel: [w409] -> w215
            tunnel: [w408] -> w212
            tunnel: [w407] -> w211
            tunnel: w180 -> [w406]
            tunnel: w178 -> [w405]
            tunnel: [w406] -> w175
            tunnel: [w405] -> w173
            tunnel: w158 -> [w401]
            tunnel: [w400] -> w155
            tunnel: w148 -> [w404]
            tunnel: [w404] -> w146
            tunnel: w374 -> [w1478]
            tunnel: [w1478] -> w373
            tunnel: w372 -> [w1477]
            tunnel: [w1477] -> w371
            tunnel: w370 -> [w1473]
            tunnel: [w1473] -> w369
            tunnel: w368 -> [w1474]
            tunnel: [w1474] -> w367
            tunnel: [w1474] -> w366
            tunnel: w365 -> [w1476]
            tunnel: [w1476] -> w364
            tunnel: w363 -> [w1475]
            tunnel: [w1475] -> w362
            tunnel: [w1474] -> w359
            tunnel: [w1474] -> w345
            tunnel: w330 -> [w1472]
            tunnel: [w1472] -> w328
            tunnel: w326 -> [w1471]
            tunnel: [w1471] -> w323
            tunnel: [w1470] -> w307
            tunnel: w306 -> [w1470]
            tunnel: [w1469] -> w304
            tunnel: w303 -> [w1469]
            tunnel: [w1468] -> w302
            tunnel: w301 -> [w1468]
            tunnel: [w1467] -> w288
            tunnel: w287 -> [w1467]
            tunnel: [w1466] -> w259
            tunnel: w258 -> [w1466]
            tunnel: [w1465] -> w241
            tunnel: w240 -> [w1465]
            tunnel: [w1464] -> w237
            tunnel: w236 -> [w1464]
            tunnel: w219 -> [w1463]
            tunnel: [w1463] -> w218
            tunnel: [w1462] -> w216
            tunnel: w215 -> [w1462]
            tunnel: [w1461] -> w214
            tunnel: w212 -> [w1461]
            tunnel: w211 -> [w1460]
            tunnel: [w1460] -> w210
            tunnel: [w1459] -> w176
            tunnel: w175 -> [w1459]
            tunnel: [w1458] -> w174
            tunnel: w173 -> [w1458]
            tunnel: [w1457] -> w156
            tunnel: w155 -> [w1457]
            tunnel: w146 -> [w1456]
            tunnel: [w1456] -> w145
            tunnel: [w1508] -> w344
            tunnel: w373 -> [w1537]
            tunnel: w371 -> [w1536]
            tunnel: w369 -> [w1533]
            tunnel: w367 -> [w1532]
            tunnel: w366 -> [w1531]
            tunnel: w364 -> [w1521]
            tunnel: w362 -> [w1520]
            tunnel: w359 -> [w1522]
            tunnel: [w1518] -> w343
            tunnel: [w1519] -> w342
            tunnel: [w1530] -> w341
            tunnel: [w1529] -> w340
            tunnel: [w1528] -> w339
            tunnel: [w1527] -> w338
            tunnel: w345 -> [w1517]
            tunnel: [w1516] -> w337
            tunnel: [w1515] -> w336
            tunnel: [w1499] -> w335
            tunnel: [w1514] -> w334
            tunnel: w328 -> [w1513]
            tunnel: [w1513] -> w327
            tunnel: [w1512] -> w324
            tunnel: w323 -> [w1512]
            tunnel: w307 -> [w1511]
            tunnel: [w1511] -> w305
            tunnel: w304 -> [w1510]
            tunnel: w302 -> [w1509]
            tunnel: [w1510] -> w300
            tunnel: [w1509] -> w299
            tunnel: w288 -> [w1507]
            tunnel: [w1503] -> w260
            tunnel: w259 -> [w1503]
            tunnel: w241 -> [w1501]
            tunnel: w237 -> [w1500]
            tunnel: [w1494] -> w235
            tunnel: [w1499] -> w234
            tunnel: [w1497] -> w233
            tunnel: [w1495] -> w232
            tunnel: w218 -> [w1498]
            tunnel: [w1498] -> w217
            tunnel: w216 -> [w1497]
            tunnel: w214 -> [w1496]
            tunnel: [w1496] -> w213
            tunnel: w210 -> [w1495]
            tunnel: [w1494] -> w188
            tunnel: [w1493] -> w185
            tunnel: w176 -> [w1492]
            tunnel: w174 -> [w1491]
            tunnel: [w1488] -> w169
            tunnel: [w1486] -> w168
            tunnel: [w1488] -> w167
            tunnel: [w1487] -> w163
            tunnel: [w1486] -> w160
            tunnel: w156 -> [w1483]
            tunnel: [w1482] -> w154
            tunnel: w145 -> [w1481]
            tunnel: [w1481] -> w144
            tunnel: [w1480] -> w142
            tunnel: [w1479] -> w133
            tunnel: w344 -> [w1782]
            tunnel: [w1779] -> w318
            tunnel: w343 -> [w1795]
            tunnel: [w1795] -> w317
            tunnel: w342 -> [w1794]
            tunnel: [w1794] -> w316
            tunnel: w341 -> [w1793]
            tunnel: [w1793] -> w315
            tunnel: w340 -> [w1792]
            tunnel: [w1792] -> w314
            tunnel: w339 -> [w1791]
            tunnel: [w1791] -> w313
            tunnel: w338 -> [w1790]
            tunnel: [w1790] -> w312
            tunnel: [w1783] -> w311
            tunnel: w337 -> [w1776]
            tunnel: w336 -> [w1784]
            tunnel: w335 -> [w1783]
            tunnel: w334 -> [w1785]
            tunnel: [w1782] -> w310
            tunnel: w327 -> [w1781]
            tunnel: w324 -> [w1780]
            tunnel: [w1778] -> w309
            tunnel: [w1766] -> w308
            tunnel: w305 -> [w1777]
            tunnel: w300 -> [w1774]
            tunnel: w299 -> [w1773]
            tunnel: [w1775] -> w296
            tunnel: [w1772] -> w293
            tunnel: [w1771] -> w290
            tunnel: [w1767] -> w289
            tunnel: [w1765] -> w261
            tunnel: w260 -> [w1765]
            tunnel: w235 -> [w1764]
            tunnel: w234 -> [w1763]
            tunnel: w233 -> [w1762]
            tunnel: w232 -> [w1760]
            tunnel: [w1758] -> w231
            tunnel: [w1757] -> w230
            tunnel: [w1756] -> w229
            tunnel: [w1755] -> w228
            tunnel: w217 -> [w1759]
            tunnel: w213 -> [w1761]
            tunnel: [w1758] -> w209
            tunnel: [w1757] -> w208
            tunnel: [w1756] -> w207
            tunnel: [w1755] -> w206
            tunnel: [w1754] -> w189
            tunnel: w188 -> [w1754]
            tunnel: [w1753] -> w186
            tunnel: w185 -> [w1753]
            tunnel: w169 -> [w1752]
            tunnel: w168 -> [w1751]
            tunnel: w167 -> [w1750]
            tunnel: [w1750] -> w166
            tunnel: [w1749] -> w164
            tunnel: w163 -> [w1749]
            tunnel: w160 -> [w1748]
            tunnel: [w1748] -> w159
            tunnel: w154 -> [w1747]
            tunnel: [w1745] -> w153
            tunnel: w144 -> [w1744]
            tunnel: [w1743] -> w143
            tunnel: w142 -> [w1743]
            tunnel: [w1742] -> w134
            tunnel: w133 -> [w1742]
            tunnel: w318 -> [w1833]
            tunnel: [w1840] -> w358
            tunnel: [w1839] -> w357
            tunnel: w317 -> [w1839]
            tunnel: [w1834] -> w354
            tunnel: w316 -> [w1834]
            tunnel: [w1838] -> w352
            tunnel: w315 -> [w1838]
            tunnel: [w1837] -> w350
            tunnel: w314 -> [w1837]
            tunnel: [w1836] -> w348
            tunnel: w313 -> [w1836]
            tunnel: [w1835] -> w346
            tunnel: w312 -> [w1835]
            tunnel: w311 -> [w1822]
            tunnel: w310 -> [w1823]
            tunnel: w309 -> [w1801]
            tunnel: [w1801] -> w321
            tunnel: w308 -> [w1824]
            tunnel: [w1824] -> w319
            tunnel: [w1826] -> w297
            tunnel: w296 -> [w1826]
            tunnel: [w1827] -> w294
            tunnel: w293 -> [w1827]
            tunnel: [w1828] -> w291
            tunnel: w290 -> [w1828]
            tunnel: w289 -> [w1832]
            tunnel: [w1821] -> w262
            tunnel: w261 -> [w1821]
            tunnel: w231 -> [w1818]
            tunnel: w230 -> [w1817]
            tunnel: w229 -> [w1816]
            tunnel: w228 -> [w1815]
            tunnel: w209 -> [w1814]
            tunnel: w208 -> [w1813]
            tunnel: w207 -> [w1812]
            tunnel: w206 -> [w1811]
            tunnel: [w1814] -> w204
            tunnel: [w1813] -> w202
            tunnel: [w1812] -> w200
            tunnel: [w1811] -> w198
            tunnel: w189 -> [w1810]
            tunnel: [w1809] -> w187
            tunnel: w186 -> [w1809]
            tunnel: w166 -> [w1806]
            tunnel: [w1805] -> w165
            tunnel: w164 -> [w1805]
            tunnel: w159 -> [w1804]
            tunnel: w153 -> [w1802]
            tunnel: [w1802] -> w150
            tunnel: w143 -> [w1800]
            tunnel: [w1800] -> w139
            tunnel: [w1799] -> w135
            tunnel: w134 -> [w1799]
            tunnel: w358 -> [w1856]
            tunnel: w357 -> [w1871]
            tunnel: w354 -> [w1865]
            tunnel: w352 -> [w1870]
            tunnel: w350 -> [w1867]
            tunnel: w348 -> [w1869]
            tunnel: w346 -> [w1868]
            tunnel: w321 -> [w1861]
            tunnel: w319 -> [w1860]
            tunnel: w297 -> [w1859]
            tunnel: w294 -> [w1858]
            tunnel: w291 -> [w1857]
            tunnel: [w1850] -> w182
            tunnel: [w1871] -> w274
            tunnel: [w1865] -> w273
            tunnel: [w1870] -> w272
            tunnel: [w1867] -> w271
            tunnel: [w1869] -> w270
            tunnel: [w1868] -> w269
            tunnel: [w1861] -> w268
            tunnel: [w1860] -> w267
            tunnel: [w1859] -> w266
            tunnel: [w1858] -> w265
            tunnel: [w1857] -> w264
            tunnel: [w1855] -> w263
            tunnel: w262 -> [w1855]
            tunnel: [w1854] -> w205
            tunnel: w204 -> [w1854]
            tunnel: [w1853] -> w203
            tunnel: w202 -> [w1853]
            tunnel: [w1852] -> w201
            tunnel: w200 -> [w1852]
            tunnel: [w1851] -> w199
            tunnel: w198 -> [w1851]
            tunnel: w187 -> [w1849]
            tunnel: [w1848] -> w172
            tunnel: [w1847] -> w171
            tunnel: w165 -> [w1846]
            tunnel: [w1845] -> w162
            tunnel: [w1844] -> w161
            tunnel: [w1843] -> w151
            tunnel: w150 -> [w1843]
            tunnel: [w1842] -> w140
            tunnel: w139 -> [w1842]
            tunnel: [w1841] -> w136
            tunnel: w135 -> [w1841]
            tunnel: w274 -> [w1921]
            tunnel: w273 -> [w1920]
            tunnel: w272 -> [w1919]
            tunnel: w271 -> [w1918]
            tunnel: w270 -> [w1917]
            tunnel: w269 -> [w1916]
            tunnel: w268 -> [w1915]
            tunnel: w267 -> [w1914]
            tunnel: w266 -> [w1913]
            tunnel: w265 -> [w1912]
            tunnel: w264 -> [w1911]
            tunnel: w263 -> [w1904]
            tunnel: [w1921] -> w256
            tunnel: [w1920] -> w255
            tunnel: [w1919] -> w254
            tunnel: [w1918] -> w253
            tunnel: [w1917] -> w252
            tunnel: [w1916] -> w251
            tunnel: [w1915] -> w250
            tunnel: [w1914] -> w249
            tunnel: [w1913] -> w248
            tunnel: [w1912] -> w247
            tunnel: [w1911] -> w246
            tunnel: [w1904] -> w245
            tunnel: [w1903] -> w244
            tunnel: w205 -> [w1901]
            tunnel: w203 -> [w1900]
            tunnel: w201 -> [w1899]
            tunnel: w199 -> [w1898]
            tunnel: [w1901] -> w197
            tunnel: [w1900] -> w195
            tunnel: [w1899] -> w193
            tunnel: [w1898] -> w191
            tunnel: w172 -> [w1897]
            tunnel: w171 -> [w1896]
            tunnel: [w1891] -> w170
            tunnel: w162 -> [w1890]
            tunnel: w161 -> [w1889]
            tunnel: [w1888] -> w152
            tunnel: w151 -> [w1888]
            tunnel: [w1887] -> w141
            tunnel: w140 -> [w1887]
            tunnel: [w1886] -> w137
            tunnel: w136 -> [w1886]
            tunnel: [w1935] -> w292
            tunnel: [w1936] -> w295
            tunnel: [w1937] -> w298
            tunnel: [w1938] -> w320
            tunnel: [w1939] -> w322
            tunnel: [w1940] -> w347
            tunnel: [w1941] -> w349
            tunnel: [w1942] -> w351
            tunnel: [w1943] -> w353
            tunnel: [w1944] -> w355
            tunnel: [w1945] -> w356
            tunnel: w256 -> [w1945]
            tunnel: w255 -> [w1944]
            tunnel: w254 -> [w1943]
            tunnel: w253 -> [w1942]
            tunnel: w252 -> [w1941]
            tunnel: w251 -> [w1940]
            tunnel: w250 -> [w1939]
            tunnel: w249 -> [w1938]
            tunnel: w248 -> [w1937]
            tunnel: w247 -> [w1936]
            tunnel: w246 -> [w1935]
            tunnel: w245 -> [w1931]
            tunnel: w244 -> [w1930]
            tunnel: [w1929] -> w196
            tunnel: w197 -> [w1929]
            tunnel: [w1928] -> w194
            tunnel: w195 -> [w1928]
            tunnel: [w1927] -> w192
            tunnel: w193 -> [w1927]
            tunnel: [w1926] -> w190
            tunnel: w191 -> [w1926]
            tunnel: [w1925] -> w184
            tunnel: w170 -> [w1925]
            tunnel: [w1924] -> w149
            tunnel: w152 -> [w1924]
            tunnel: w141 -> [w1923]
            tunnel: [w1923] -> w138
            tunnel: w137 -> [w1922]
            tunnel: [w1922] -> w132
            frame #0 {
              n18 = Tick Count (ms)() -> (millisecond timer value=w388:u32)
            }
            frame #1 {
              n19 = while {
                tunnel: w425 -> [w435]
                tunnel: [w434] -> w424
                tunnel: [w430] -> w423
                tunnel: w411 -> [w432]
                tunnel: w401 -> [w431]
                tunnel: [w429] -> w403
                tunnel: [w428] -> w402
                stop <- w436 stop-if-true
                n20 = event shown="[15] \"Get Values\": Value Change" {
                  selector: _ -> [_ _ _ _ _ _ _ _ _ _ _ _ _ _ _ _ _ _ _ _ _]
                  dyn-events: _ -> [_ _ _ _ _ _ _ _ _ _ _ _ _ _ _ _ _ _ _ _ _]
                  timeout: 1 -> [_ _ _ _ _ _ _ _ _ _ _ _ _ _ _ _ _ _ _ _ _]
                  tunnel: [TRUE ("Set Gauge to Zero") w450 w501 w552 w577 w601 w630 w659 w698 w736 w794 w853 w907 w961 w1043 w1125 w1199 w1273 w1347 "Set Gauge to Zero" _] -> w436
                  tunnel: w435 -> [w443 w449 w496 w549 w571 w599 w627 w655 w693 w735 w789 w849 w905 w959 w1041 w1123 w1195 w1271 w1345 w1425 w1450]
                  tunnel: [w442 w448 w495 w548 w570 w598 w624 w657 w692 w733 w791 w851 w904 w958 w1040 w1122 w1197 w1270 w1344 w1424 w1449] -> w434
                  tunnel: [w441 w447 w494 w547 w569 w597 w623 w656 w691 w734 w790 w850 w903 w957 w1039 w1121 w1196 w1269 w1343 w1423 w1448] -> w430
                  tunnel: w432 -> [_ _ _ _ _ _ _ _ _ _ _ _ _ _ _ _ _ _ _ w1421 _]
                  tunnel: w431 -> [w439 w446 w499 w546 w574 w596 w628 w652 w696 w732 w788 w848 w902 w956 w1036 w1120 w1194 w1268 w1342 w1416 w1442]
                  tunnel: [w437 w445 w498 w545 w573 w595 w626 w654 w695 w731 w793 w847 w901 w955 w1038 w1119 w1193 w1267 w1341 w1415 w1441] -> w429
                  tunnel: [w438 w444 w497 w544 w572 w594 w625 w653 w694 w730 w792 w846 w900 w954 w1037 w1118 w1192 w1266 w1340 w1414 w1440] -> w428
                  event Timeout {
                    n21 = event-data() -> ()  [unwired: 1 in, 1 out]
                    n22 = Unbundle(w443) -> ("VISA resource name out"=w442:refnum<visa-resource-name>, "error out"=w441:errorcluster)  [unwired: 2 out]
                    n23 = Unbundle(w439) -> ("VISA resource name out"=w437:refnum<visa-resource-name>, "error out"=w438:errorcluster)  [unwired: 2 out]
                  }
                  event "Setpoint\n START": Value Change {
                    n24 = event-data() -> ()  [unwired: 1 in, 1 out]
                    n25 = stacked-sequence {
                      tunnel: w449 -> [_ w456 _]
                      tunnel: [_ w455 _] -> w447
                      tunnel: [_ w454 _] -> w448
                      frame #0 {
                        n26 = property on="Setpoint\n START" class="Bool"("Blinking"=TRUE) -> ()  [unwired: 2 in, 2 out]
                        n27 = property on="ON" class="Bool (strict)"("Blinking"=FALSE) -> ()  [unwired: 2 in, 2 out]
                      }
                      frame #1 {
                        n28 = for {
                          N: 2 -> [_]
                          tunnel: w456 -> [w460]
                          tunnel: [w459] -> w455
                          tunnel: [w458] -> w454
                          i -> [w462]
                          n29 = flat-sequence {
                            tunnel: [w465] -> w461
                            tunnel: w462 -> [w464]
                            tunnel: [w483] -> w463
                            tunnel: w461 -> [w482]
                            tunnel: w460 -> [w484]
                            tunnel: [w481] -> w459
                            tunnel: [w480] -> w458
                            tunnel: w463 -> [w490]
                            tunnel: w462 -> [w489]
                            frame #0 {
                              n30 = case shown="0, Default" w464 {
                                tunnel: [w474 w476] -> w465
                                frame 0, Default {
                                n31 = Multiply(x=10.0, y="SP 1 input (°C)") -> (x*y=w471:dbl)
                                n32 = local read "RAM"() -> (w469:bool)
                                n33 = Number To Hexadecimal String(1:i16 5 ("width (-)"), 2:w471) -> (0:w473:string)
                                n34 = Select(t="*P012", s=w469, f="*P012") -> (s? t:f=w466:string)
                                n35 = Concatenate Strings(w466, w473) -> (w474:string)
                                }
                                frame 1 {
                                n36 = local read "RAM"() -> (w479:bool)
                                n37 = Select(t="*G01", s=w479, f="*R01") -> (s? t:f=w476:string)
                                }
                              }
                            }
                            frame #1 {
                              n38 = Unbundle(w484) -> ("VISA resource name out"=w485:refnum<visa-resource-name>, "error out"=w487:errorcluster, "Delay (ms)"=w486:u32, "Write/\nRead"=w488:bool)
                              n39 = call "I3252_Comm_Interface.vi"("VISA resource name in"=w485, "error in"=w487, "Delay (ms)"=w486, "Write"=w488, "String to Write"=w482, "Read"=w488) -> ("VISA resource name out"=w480:refnum<visa-resource-name>, "error out"=w481:errorcluster, "Read String"=w483:string)  [unwired: 2 in]
                            }
                            frame #2 {
                              n40 = case shown="0, Default" w489 {
                                tunnel: w490 -> [_ w492]
                                frame 0, Default {
                                }
                                frame 1 {
                                n41 = call "I3252_Edit_Setpoint.vi"("Read String"=w492) -> ("Setpoint is"=→"SP 1 is (°C)":dbl)
                                }
                              }
                            }
                          }
                        }
                      }
                      frame #2 {
                        n42 = property on="Setpoint\n START" class="Bool"("Blinking"=FALSE) -> ()  [unwired: 2 in, 2 out]
                      }
                    }
                    n43 = Unbundle(w446) -> ("VISA resource name out"=w445:refnum<visa-resource-name>, "error out"=w444:errorcluster)  [unwired: 2 out]
                    n44 = Not(x="Setpoint\n START") -> (.not. x?=w450:bool)
                  }
                  event "Setpoint\n START\n2": Value Change {
                    n45 = event-data() -> ()  [unwired: 1 in, 1 out]
                    n46 = stacked-sequence {
                      tunnel: w499 -> [_ w506 _]
                      tunnel: [_ w505 _] -> w497
                      tunnel: [_ w504 _] -> w498
                      frame #0 {
                        n47 = property on="Setpoint\n START\n2" class="Bool"("Blinking"=TRUE) -> ()  [unwired: 2 in, 2 out]
                        n48 = property on="ON 2" class="Bool (strict)"("Blinking"=FALSE) -> ()  [unwired: 2 in, 2 out]
                      }
                      frame #1 {
                        n49 = for {
                          N: 2 -> [_]
                          tunnel: w506 -> [w510]
                          tunnel: [w509] -> w505
                          tunnel: [w508] -> w504
                          i -> [w512]
                          n50 = flat-sequence {
                            tunnel: [w515] -> w511
                            tunnel: w512 -> [w514]
                            tunnel: [w533] -> w513
                            tunnel: w511 -> [w532]
                            tunnel: w510 -> [w534]
                            tunnel: [w531] -> w509
                            tunnel: [w530] -> w508
                            tunnel: w513 -> [w540]
                            tunnel: w512 -> [w539]
                            frame #0 {
                              n51 = case shown="0, Default" w514 {
                                tunnel: [w524 w526] -> w515
                                frame 0, Default {
                                n52 = Multiply(x=10.0, y="SP 2 input (°C)") -> (x*y=w522:dbl)
                                n53 = local read "RAM"() -> (w520:bool)
                                n54 = Number To Hexadecimal String(1:i16 5 ("width (-)"), 2:w522) -> (0:w523:string)
                                n55 = Select(t="*P012", s=w520, f="*P012") -> (s? t:f=w517:string)
                                n56 = Concatenate Strings(w517, w523) -> (w524:string)
                                }
                                frame 1 {
                                n57 = local read "RAM"() -> (w529:bool)
                                n58 = Select(t="*G01", s=w529, f="*R01") -> (s? t:f=w526:string)
                                }
                              }
                            }
                            frame #1 {
                              n59 = Unbundle(w534) -> ("VISA resource name out"=w535:refnum<visa-resource-name>, "error out"=w537:errorcluster, "Delay (ms) 2"=w536:u32, "Write/\nRead \n\n2"=w538:bool)
                              n60 = call "I3252_Comm_Interface.vi"("VISA resource name in"=w535, "error in"=w537, "Delay (ms)"=w536, "Write"=w538, "String to Write"=w532, "Read"=w538) -> ("VISA resource name out"=w530:refnum<visa-resource-name>, "error out"=w531:errorcluster, "Read String"=w533:string)  [unwired: 2 in]
                            }
                            frame #2 {
                              n61 = case shown="1" w539 {
                                tunnel: w540 -> [_ w542]
                                frame 0, Default {
                                }
                                frame 1 {
                                n62 = call "I3252_Edit_Setpoint.vi"("Read String"=w542) -> ("Setpoint is"=→"SP 2 is (°C)":dbl)
                                }
                              }
                            }
                          }
                        }
                      }
                      frame #2 {
                        n63 = property on="Setpoint\n START\n2" class="Bool"("Blinking"=FALSE) -> ()  [unwired: 2 in, 2 out]
                      }
                    }
                    n64 = Not(x="Setpoint\n START\n2") -> (.not. x?=w501:bool)
                    n65 = Unbundle(w496) -> ("VISA resource name out"=w495:refnum<visa-resource-name>, "error out"=w494:errorcluster)  [unwired: 2 out]
                  }
                  event "Standby": Value Change {
                    n66 = event-data() -> ()  [unwired: 1 in, 1 out]
                    n67 = flat-sequence {
                      tunnel: [w560] -> w550
                      tunnel: w550 -> [w564]
                      tunnel: w549 -> [w563]
                      tunnel: [w562] -> w547
                      tunnel: [w561] -> w548
                      frame #0 {
                        n68 = local read "Standby"() -> (w553:bool)
                        n69 = Select(t=TRUE, s=w553, f=FALSE) -> (s? t:f=w556:bool)
                        n70 = property on="Standby" class="Bool (strict)"("Blinking"=w556) -> ()  [unwired: 2 in, 2 out]
                      }
                      frame #1 {
                        n71 = local read "Standby"() -> (w558:bool)
                        n72 = Select(t="*D03", s=w558, f="*E03") -> (s? t:f=w560:string)
                      }
                      frame #2 {
                        n73 = Unbundle(w563) -> ("VISA resource name out"=w565:refnum<visa-resource-name>, "error out"=w567:errorcluster, "Delay (ms)"=w566:u32, "Write/\nRead"=w568:bool)
                        n74 = call "I3252_Comm_Interface.vi"("VISA resource name in"=w565, "error in"=w567, "Delay (ms)"=w566, "Write"=w568, "String to Write"=w564, "Read"=w568) -> ("VISA resource name out"=w561:refnum<visa-resource-name>, "error out"=w562:errorcluster)  [unwired: 2 in, 1 out]
                      }
                    }
                    n75 = Not(x="Standby") -> (.not. x?=w552:bool)
                    n76 = Unbundle(w546) -> ("VISA resource name out"=w545:refnum<visa-resource-name>, "error out"=w544:errorcluster)  [unwired: 2 out]
                  }
                  event "Standby\n2": Value Change {
                    n77 = event-data() -> ()  [unwired: 1 in, 1 out]
                    n78 = flat-sequence {
                      tunnel: [w585] -> w576
                      tunnel: w576 -> [w589]
                      tunnel: w574 -> [w588]
                      tunnel: [w587] -> w572
                      tunnel: [w586] -> w573
                      frame #0 {
                        n79 = local read "Standby\n2"() -> (w579:bool)
                        n80 = Select(t=TRUE, s=w579, f=FALSE) -> (s? t:f=w578:bool)
                        n81 = property on="Standby\n2" class="Bool (strict)"("Blinking"=w578) -> ()  [unwired: 2 in, 2 out]
                      }
                      frame #1 {
                        n82 = local read "Standby\n2"() -> (w583:bool)
                        n83 = Select(t="*D03", s=w583, f="*E03") -> (s? t:f=w585:string)
                      }
                      frame #2 {
                        n84 = Unbundle(w588) -> ("VISA resource name out"=w590:refnum<visa-resource-name>, "error out"=w592:errorcluster, "Delay (ms) 2"=w591:u32, "Write/\nRead \n\n2"=w593:bool)
                        n85 = call "I3252_Comm_Interface.vi"("VISA resource name in"=w590, "error in"=w592, "Delay (ms)"=w591, "Write"=w593, "String to Write"=w589, "Read"=w593) -> ("VISA resource name out"=w586:refnum<visa-resource-name>, "error out"=w587:errorcluster)  [unwired: 2 in, 1 out]
                      }
                    }
                    n86 = Not(x="Standby\n2") -> (.not. x?=w577:bool)
                    n87 = Unbundle(w571) -> ("VISA resource name out"=w570:refnum<visa-resource-name>, "error out"=w569:errorcluster)  [unwired: 2 out]
                  }
                  event "Set Command": Value Change {
                    n88 = event-data() -> ()  [unwired: 1 in, 1 out]
                    n89 = stacked-sequence {
                      tunnel: w599 -> [_ w606 _]
                      tunnel: [_ w605 _] -> w598
                      tunnel: [_ w604 _] -> w597
                      frame #0 {
                        n90 = property on="Set Command" class="Bool"("Blinking"=TRUE) -> ()  [unwired: 2 in, 2 out]
                        n91 = property on="ON" class="Bool (strict)"("Blinking"=FALSE) -> ()  [unwired: 2 in, 2 out]
                      }
                      frame #1 {
                        n92 = flat-sequence {
                          tunnel: [w611] -> w608
                          tunnel: [w614] -> w607
                          tunnel: w608 -> [w615]
                          tunnel: w606 -> [w616]
                          tunnel: [w613] -> w605
                          tunnel: [w612] -> w604
                          tunnel: w607 -> [w621]
                          frame #0 {
                            n93 = Concatenate Strings("*", "Command input") -> (w611:string)
                          }
                          frame #1 {
                            n94 = Unbundle(w616) -> ("VISA resource name out"=w620:refnum<visa-resource-name>, "error out"=w618:errorcluster, "Delay (ms)"=w619:u32, "Write/\nRead"=w617:bool)
                            n95 = call "I3252_Comm_Interface.vi"("VISA resource name in"=w620, "error in"=w618, "Delay (ms)"=w619, "Write"=w617, "String to Write"=w615, "Read"=w617) -> ("VISA resource name out"=w613:refnum<visa-resource-name>, "error out"=w612:errorcluster, "Read String"=w614:string)  [unwired: 2 in]
                          }
                          frame #2 {
                            "Command output" <- w621
                          }
                        }
                      }
                      frame #2 {
                        n96 = property on="Set Command" class="Bool"("Blinking"=FALSE) -> ()  [unwired: 2 in, 2 out]
                      }
                    }
                    n97 = Not(x="Set Command") -> (.not. x?=w601:bool)
                    n98 = Unbundle(w596) -> ("VISA resource name out"=w595:refnum<visa-resource-name>, "error out"=w594:errorcluster)  [unwired: 2 out]
                  }
                  event "Set Command\n\n 2": Value Change {
                    n99 = event-data() -> ()  [unwired: 1 in, 1 out]
                    n100 = stacked-sequence {
                      tunnel: w628 -> [_ w635 _]
                      tunnel: [_ w634 _] -> w626
                      tunnel: [_ w633 _] -> w625
                      frame #0 {
                        n101 = property on="Set Command\n\n 2" class="Bool"("Blinking"=TRUE) -> ()  [unwired: 2 in, 2 out]
                        n102 = property on="ON 2" class="Bool (strict)"("Blinking"=FALSE) -> ()  [unwired: 2 in, 2 out]
                      }
                      frame #1 {
                        n103 = flat-sequence {
                          tunnel: [w640] -> w637
                          tunnel: [w643] -> w636
                          tunnel: w637 -> [w644]
                          tunnel: w635 -> [w645]
                          tunnel: [w642] -> w634
                          tunnel: [w641] -> w633
                          tunnel: w636 -> [w650]
                          frame #0 {
                            n104 = Concatenate Strings("*", "Command input 2") -> (w640:string)
                          }
                          frame #1 {
                            n105 = Unbundle(w645) -> ("VISA resource name out"=w649:refnum<visa-resource-name>, "error out"=w647:errorcluster, "Delay (ms) 2"=w648:u32, "Write/\nRead \n\n2"=w646:bool)
                            n106 = call "I3252_Comm_Interface.vi"("VISA resource name in"=w649, "error in"=w647, "Delay (ms)"=w648, "Write"=w646, "String to Write"=w644, "Read"=w646) -> ("VISA resource name out"=w642:refnum<visa-resource-name>, "error out"=w641:errorcluster, "Read String"=w643:string)  [unwired: 2 in]
                          }
                          frame #2 {
                            "Command output 2" <- w650
                          }
                        }
                      }
                      frame #2 {
                        n107 = property on="Set Command\n\n 2" class="Bool"("Blinking"=FALSE) -> ()  [unwired: 2 in, 2 out]
                      }
                    }
                    n108 = Not(x="Set Command\n\n 2") -> (.not. x?=w630:bool)
                    n109 = Unbundle(w627) -> ("VISA resource name out"=w624:refnum<visa-resource-name>, "error out"=w623:errorcluster)  [unwired: 2 out]
                  }
                  event "Reset\nSTOP": Value Change {
                    n110 = event-data() -> ()  [unwired: 1 in, 1 out]
                    n111 = stacked-sequence {
                      tunnel: [_ w666 _] -> w656
                      tunnel: [_ w665 _] -> w657
                      tunnel: w655 -> [_ w663 _]
                      frame #0 {
                        n112 = property on="Reset\nSTOP" class="Bool"("Blinking"=TRUE) -> ()  [unwired: 2 in, 2 out]
                        n113 = property on="ON" class="Bool (strict)"("Blinking"=FALSE) -> ()  [unwired: 2 in, 2 out]
                      }
                      frame #1 {
                        n114 = for {
                          N: 2 -> [_]
                          tunnel: [w672] -> w666
                          tunnel: [w671] -> w665
                          tunnel: w663 -> [w670]
                          i -> [w668]
                          n115 = flat-sequence {
                            tunnel: w668 -> [w674]
                            tunnel: [w673] -> w669
                            tunnel: [w679] -> w672
                            tunnel: [w680] -> w671
                            tunnel: w670 -> [w681]
                            tunnel: w669 -> [w678]
                            tunnel: [w677] -> w667
                            tunnel: w668 -> [w687]
                            tunnel: w667 -> [w686]
                            frame #0 {
                              n116 = case shown="0, Default" w674 {
                                tunnel: ["*Z02" "*G01"] -> w673
                                frame 0, Default {
                                }
                                frame 1 {
                                }
                              }
                            }
                            frame #1 {
                              n117 = Unbundle(w681) -> ("VISA resource name out"=w682:refnum<visa-resource-name>, "error out"=w684:errorcluster, "Delay (ms)"=w683:u32, "Write/\nRead"=w685:bool)
                              n118 = call "I3252_Comm_Interface.vi"("VISA resource name in"=w682, "error in"=w684, "Delay (ms)"=w683, "Write"=w685, "String to Write"=w678, "Read"=w685) -> ("VISA resource name out"=w680:refnum<visa-resource-name>, "error out"=w679:errorcluster, "Read String"=w677:string)  [unwired: 2 in]
                            }
                            frame #2 {
                              n119 = case shown="0, Default" w687 {
                                tunnel: w686 -> [_ w689]
                                frame 0, Default {
                                }
                                frame 1 {
                                n120 = call "I3252_Edit_Setpoint.vi"("Read String"=w689) -> ("Setpoint is"=w688:dbl)
                                n121 = local write "SP 1 is (°C)"(w688) -> ()
                                }
                              }
                            }
                          }
                        }
                        n122 = Wait (ms)(milliseconds to wait=u32 4000) -> ()  [unwired: 1 out]
                      }
                      frame #2 {
                        n123 = property on="Reset\nSTOP" class="Bool"("Blinking"=FALSE) -> ()  [unwired: 2 in, 2 out]
                      }
                    }
                    n124 = Not(x="Reset\nSTOP") -> (.not. x?=w659:bool)
                    n125 = Unbundle(w652) -> ("VISA resource name out"=w654:refnum<visa-resource-name>, "error out"=w653:errorcluster)  [unwired: 2 out]
                  }
                  event "Reset\nSTOP 2": Value Change {
                    n126 = event-data() -> ()  [unwired: 1 in, 1 out]
                    n127 = stacked-sequence {
                      tunnel: [_ w705 _] -> w694
                      tunnel: [_ w704 _] -> w695
                      tunnel: w696 -> [_ w702 _]
                      frame #0 {
                        n128 = property on="Reset\nSTOP 2" class="Bool"("Blinking"=TRUE) -> ()  [unwired: 2 in, 2 out]
                        n129 = property on="ON 2" class="Bool (strict)"("Blinking"=FALSE) -> ()  [unwired: 2 in, 2 out]
                      }
                      frame #1 {
                        n130 = for {
                          N: 2 -> [_]
                          tunnel: [w711] -> w705
                          tunnel: [w710] -> w704
                          tunnel: w702 -> [w709]
                          i -> [w707]
                          n131 = flat-sequence {
                            tunnel: w707 -> [w713]
                            tunnel: [w712] -> w708
                            tunnel: [w718] -> w711
                            tunnel: [w719] -> w710
                            tunnel: w709 -> [w720]
                            tunnel: w708 -> [w717]
                            tunnel: [w716] -> w706
                            tunnel: w707 -> [w726]
                            tunnel: w706 -> [w725]
                            frame #0 {
                              n132 = case shown="0, Default" w713 {
                                tunnel: ["*Z02" "*G01"] -> w712
                                frame 0, Default {
                                }
                                frame 1 {
                                }
                              }
                            }
                            frame #1 {
                              n133 = Unbundle(w720) -> ("VISA resource name out"=w721:refnum<visa-resource-name>, "error out"=w723:errorcluster, "Delay (ms) 2"=w722:u32, "Write/\nRead \n\n2"=w724:bool)
                              n134 = call "I3252_Comm_Interface.vi"("VISA resource name in"=w721, "error in"=w723, "Delay (ms)"=w722, "Write"=w724, "String to Write"=w717, "Read"=w724) -> ("VISA resource name out"=w719:refnum<visa-resource-name>, "error out"=w718:errorcluster, "Read String"=w716:string)  [unwired: 2 in]
                            }
                            frame #2 {
                              n135 = case shown="1" w726 {
                                tunnel: w725 -> [_ w728]
                                frame 0, Default {
                                }
                                frame 1 {
                                n136 = call "I3252_Edit_Setpoint.vi"("Read String"=w728) -> ("Setpoint is"=w727:dbl)
                                n137 = local write "SP 2 is (°C)"(w727) -> ()
                                }
                              }
                            }
                          }
                        }
                        n138 = Wait (ms)(milliseconds to wait=u32 4000) -> ()  [unwired: 1 out]
                      }
                      frame #2 {
                        n139 = property on="Reset\nSTOP 2" class="Bool"("Blinking"=FALSE) -> ()  [unwired: 2 in, 2 out]
                      }
                    }
                    n140 = Not(x="Reset\nSTOP 2") -> (.not. x?=w698:bool)
                    n141 = Unbundle(w693) -> ("VISA resource name out"=w692:refnum<visa-resource-name>, "error out"=w691:errorcluster)  [unwired: 2 out]
                  }
                  event "Auto Tune": Value Change {
                    n142 = event-data() -> ()  [unwired: 1 in, 1 out]
                    n143 = stacked-sequence {
                      tunnel: w735 -> [_ w742 w787]
                      tunnel: [_ w741 _] -> w734
                      tunnel: [_ w740 _] -> w733
                      frame #0 {
                        n144 = property on="Auto Tune" class="Bool"("Blinking"=TRUE) -> ()  [unwired: 2 in, 2 out]
                        n145 = property on="ON" class="Bool (strict)"("Blinking"=FALSE) -> ()  [unwired: 2 in, 2 out]
                      }
                      frame #1 {
                        n146 = for {
                          N: 4 -> [_]
                          tunnel: [w747] -> w740
                          tunnel: [w746] -> w741
                          tunnel: w742 -> [w745]
                          i -> [w750]
                          n147 = flat-sequence {
                            tunnel: w750 -> [w752]
                            tunnel: [w751] -> w748
                            tunnel: w748 -> [w767]
                            tunnel: [w766] -> w749
                            tunnel: [w769] -> w747
                            tunnel: [w768] -> w746
                            tunnel: w745 -> [w765]
                            tunnel: w750 -> [w775]
                            tunnel: w749 -> [w774]
                            frame #0 {
                              n148 = case shown="0, Default" w752 {
                                tunnel: ["*V01" w755 "*W0C35" "*Z02"] -> w751
                                frame 0, Default {
                                }
                                frame 1 {
                                n149 = local read "(°C)"() -> (w754:dbl)
                                n150 = Add(x=20.0, y=w754) -> (x+y=w761:dbl)
                                n151 = Multiply(x=10.0, y=w761) -> (x*y=w758:dbl)
                                n152 = Number To Hexadecimal String(1:i16 5 ("width (-)"), 2:w758) -> (0:w757:string)
                                n153 = Concatenate Strings("*W012", w757) -> (w755:string)
                                }
                                frame 2 {
                                # "35 hex = \n00110101 bin"
                                }
                                frame 3 {
                                }
                              }
                            }
                            frame #1 {
                              n154 = Unbundle(w765) -> ("VISA resource name out"=w773:refnum<visa-resource-name>, "error out"=w771:errorcluster, "Delay (ms)"=w772:u32, "Write/\nRead"=w770:bool)
                              n155 = call "I3252_Comm_Interface.vi"("VISA resource name in"=w773, "error in"=w771, "Delay (ms)"=w772, "Write"=w770, "String to Write"=w767, "Read"=w770) -> ("VISA resource name out"=w769:refnum<visa-resource-name>, "error out"=w768:errorcluster, "Read String"=w766:string)  [unwired: 2 in]
                            }
                            frame #2 {
                              n156 = case shown="0, Default" w775 {
                                tunnel: w774 -> [w777]
                                frame 0, Default {
                                n157 = call <vilib>:"Space Constant.vi"() -> ("String"=w780:string)
                                n158 = Search/Split String(string=w777, search string/char (-)=w780) -> (match + rest of string=w779:string)  [unwired: 1 in, 2 out]
                                n159 = Fract/Exp String To Number(use system decimal point (T)=FALSE, string=w779) -> (number=w776:dbl)  [unwired: 2 in, 1 out]
                                n160 = local write "(°C)"(w776) -> ()
                                }
                              }
                            }
                          }
                        }
                        n161 = Wait (ms)(milliseconds to wait=u32 45000) -> ()  [unwired: 1 out]
                      }
                      frame #2 {
                        n162 = Unbundle(w787) -> ("VISA resource name out"=w786:refnum<visa-resource-name>, "error out"=w784:errorcluster, "Delay (ms)"=w785:u32, "Write/\nRead"=w783:bool)
                        n163 = property on="Auto Tune" class="Bool"("Blinking"=FALSE) -> ()  [unwired: 2 in, 2 out]
                        n164 = call "I3252_Comm_Interface.vi"("VISA resource name in"=w786, "error in"=w784, "Delay (ms)"=w785, "Write"=w783, "String to Write"="*W01200000", "Read"=w783) -> ()  [unwired: 2 in, 3 out]
                      }
                    }
                    n165 = Not(x="Auto Tune") -> (.not. x?=w736:bool)
                    n166 = Unbundle(w732) -> ("VISA resource name out"=w731:refnum<visa-resource-name>, "error out"=w730:errorcluster)  [unwired: 2 out]
                  }
                  event "Auto Tune 2": Value Change {
                    n167 = event-data() -> ()  [unwired: 1 in, 1 out]
                    n168 = stacked-sequence {
                      tunnel: w788 -> [_ w800 w845]
                      tunnel: [_ w799 _] -> w792
                      tunnel: [_ w798 _] -> w793
                      frame #0 {
                        n169 = property on="Auto Tune 2" class="Bool"("Blinking"=TRUE) -> ()  [unwired: 2 in, 2 out]
                        n170 = property on="ON" class="Bool (strict)"("Blinking"=FALSE) -> ()  [unwired: 2 in, 2 out]
                      }
                      frame #1 {
                        n171 = for {
                          N: 4 -> [_]
                          tunnel: [w805] -> w798
                          tunnel: [w804] -> w799
                          tunnel: w800 -> [w803]
                          i -> [w808]
                          n172 = flat-sequence {
                            tunnel: w808 -> [w810]
                            tunnel: [w809] -> w806
                            tunnel: w806 -> [w825]
                            tunnel: [w824] -> w807
                            tunnel: [w827] -> w805
                            tunnel: [w826] -> w804
                            tunnel: w803 -> [w823]
                            tunnel: w808 -> [w833]
                            tunnel: w807 -> [w832]
                            frame #0 {
                              n173 = case shown="1" w810 {
                                tunnel: ["*V01" w813 "*W0C35" "*Z02"] -> w809
                                frame 0, Default {
                                }
                                frame 1 {
                                n174 = local read "(°C) 2"() -> (w812:dbl)
                                n175 = Add(x=20.0, y=w812) -> (x+y=w819:dbl)
                                n176 = Multiply(x=10.0, y=w819) -> (x*y=w816:dbl)
                                n177 = Number To Hexadecimal String(1:i16 5 ("width (-)"), 2:w816) -> (0:w815:string)
                                n178 = Concatenate Strings("*W012", w815) -> (w813:string)
                                }
                                frame 2 {
                                # "35 hex = \n00110101 bin"
                                }
                                frame 3 {
                                }
                              }
                            }
                            frame #1 {
                              n179 = Unbundle(w823) -> ("VISA resource name out"=w831:refnum<visa-resource-name>, "error out"=w829:errorcluster, "Delay (ms) 2"=w830:u32, "Write/\nRead \n\n2"=w828:bool)
                              n180 = call "I3252_Comm_Interface.vi"("VISA resource name in"=w831, "error in"=w829, "Delay (ms)"=w830, "Write"=w828, "String to Write"=w825, "Read"=w828) -> ("VISA resource name out"=w827:refnum<visa-resource-name>, "error out"=w826:errorcluster, "Read String"=w824:string)  [unwired: 2 in]
                            }
                            frame #2 {
                              n181 = case shown="0, Default" w833 {
                                tunnel: w832 -> [w835]
                                frame 0, Default {
                                n182 = call <vilib>:"Space Constant.vi"() -> ("String"=w838:string)
                                n183 = Search/Split String(string=w835, search string/char (-)=w838) -> (match + rest of string=w837:string)  [unwired: 1 in, 2 out]
                                n184 = Fract/Exp String To Number(use system decimal point (T)=FALSE, string=w837) -> (number=w834:dbl)  [unwired: 2 in, 1 out]
                                n185 = local write "(°C) 2"(w834) -> ()
                                }
                              }
                            }
                          }
                        }
                        n186 = Wait (ms)(milliseconds to wait=u32 45000) -> ()  [unwired: 1 out]
                      }
                      frame #2 {
                        n187 = Unbundle(w845) -> ("VISA resource name out"=w844:refnum<visa-resource-name>, "error out"=w842:errorcluster, "Delay (ms) 2"=w843:u32, "Write/\nRead \n\n2"=w841:bool)
                        n188 = property on="Auto Tune 2" class="Bool"("Blinking"=FALSE) -> ()  [unwired: 2 in, 2 out]
                        n189 = call "I3252_Comm_Interface.vi"("VISA resource name in"=w844, "error in"=w842, "Delay (ms)"=w843, "Write"=w841, "String to Write"="*W01200000", "Read"=w841) -> ()  [unwired: 2 in, 3 out]
                      }
                    }
                    n190 = Not(x="Auto Tune 2") -> (.not. x?=w794:bool)
                    n191 = Unbundle(w789) -> ("VISA resource name out"=w791:refnum<visa-resource-name>, "error out"=w790:errorcluster)  [unwired: 2 out]
                  }
                  event "Write LOW/HI": Value Change {
                    n192 = event-data() -> ()  [unwired: 1 in, 1 out]
                    n193 = stacked-sequence {
                      tunnel: [_ w858 _] -> w851
                      tunnel: [_ w857 _] -> w850
                      tunnel: w849 -> [_ w856 _]
                      frame #0 {
                        n194 = property on="Write LOW/HI" class="Bool"("Blinking"=TRUE) -> ()  [unwired: 2 in, 2 out]
                        n195 = property on="ON" class="Bool (strict)"("Blinking"=FALSE) -> ()  [unwired: 2 in, 2 out]
                      }
                      frame #1 {
                        n196 = for {
                          N: 4 -> [_]
                          tunnel: [w862] -> w858
                          tunnel: [w861] -> w857
                          tunnel: w856 -> [w860]
                          i -> [w864]
                          n197 = flat-sequence {
                            tunnel: w864 -> [w866]
                            tunnel: [w867] -> w863
                            tunnel: w863 -> [w881]
                            tunnel: [w882] -> w865
                            tunnel: [w884] -> w862
                            tunnel: [w883] -> w861
                            tunnel: w860 -> [w880]
                            tunnel: w865 -> [w890]
                            tunnel: w864 -> [w889]
                            frame #0 {
                              n198 = case shown="0, Default" w866 {
                                tunnel: [w869 w875 "*R27" "*R28"] -> w867
                                frame 0, Default {
                                n199 = Number To Hexadecimal String(1:i16 2 ("width (-)"), 2:"% LOW Sollwert") -> (0:w870:string)
                                n200 = Concatenate Strings("*W27", w870) -> (w869:string)
                                }
                                frame 1 {
                                n201 = Number To Hexadecimal String(1:i16 2 ("width (-)"), 2:"% High Sollwert") -> (0:w876:string)
                                n202 = Concatenate Strings("*W28", w876) -> (w875:string)
                                }
                                frame 2 {
                                }
                                frame 3 {
                                }
                              }
                            }
                            frame #1 {
                              n203 = Unbundle(w880) -> ("VISA resource name out"=w888:refnum<visa-resource-name>, "error out"=w886:errorcluster, "Delay (ms)"=w887:u32, "Write/\nRead"=w885:bool)
                              n204 = call "I3252_Comm_Interface.vi"("VISA resource name in"=w888, "error in"=w886, "Delay (ms)"=w887, "Write"=w885, "String to Write"=w881, "Read"=w885) -> ("VISA resource name out"=w884:refnum<visa-resource-name>, "error out"=w883:errorcluster, "Read String"=w882:string)  [unwired: 2 in]
                            }
                            frame #2 {
                              n205 = case shown="0, Default" w889 {
                                tunnel: w890 -> [_ w894 w898]
                                frame 0, Default {
                                }
                                frame 2 {
                                n206 = String Subset(string=w894, offset (0)=3) -> (substring=w892:string)  [unwired: 1 in]
                                n207 = Hexadecimal String To Number(string=w892) -> (number=→"% LOW Istwert":u32)  [unwired: 2 in, 1 out]
                                }
                                frame 3 {
                                n208 = String Subset(string=w898, offset (0)=3) -> (substring=w896:string)  [unwired: 1 in]
                                n209 = Hexadecimal String To Number(string=w896) -> (number=→"% HIGH Istwert":u32)  [unwired: 2 in, 1 out]
                                }
                              }
                            }
                          }
                        }
                      }
                      frame #2 {
                        n210 = property on="Write LOW/HI" class="Bool"("Blinking"=FALSE) -> ()  [unwired: 2 in, 2 out]
                      }
                    }
                    n211 = Not(x="Write LOW/HI") -> (.not. x?=w853:bool)
                    n212 = Unbundle(w848) -> ("VISA resource name out"=w847:refnum<visa-resource-name>, "error out"=w846:errorcluster)  [unwired: 2 out]
                  }
                  event "Write LOW/HI 2": Value Change {
                    n213 = event-data() -> ()  [unwired: 1 in, 1 out]
                    n214 = stacked-sequence {
                      tunnel: [_ w912 _] -> w901
                      tunnel: [_ w911 _] -> w900
                      tunnel: w902 -> [_ w910 _]
                      frame #0 {
                        n215 = property on="Write LOW/HI 2" class="Bool"("Blinking"=TRUE) -> ()  [unwired: 2 in, 2 out]
                        n216 = property on="ON 2" class="Bool (strict)"("Blinking"=FALSE) -> ()  [unwired: 2 in, 2 out]
                      }
                      frame #1 {
                        n217 = for {
                          N: 4 -> [_]
                          tunnel: [w916] -> w912
                          tunnel: [w915] -> w911
                          tunnel: w910 -> [w914]
                          i -> [w918]
                          n218 = flat-sequence {
                            tunnel: w918 -> [w920]
                            tunnel: [w921] -> w917
                            tunnel: w917 -> [w935]
                            tunnel: [w936] -> w919
                            tunnel: [w938] -> w916
                            tunnel: [w937] -> w915
                            tunnel: w914 -> [w934]
                            tunnel: w919 -> [w944]
                            tunnel: w918 -> [w943]
                            frame #0 {
                              n219 = case shown="0, Default" w920 {
                                tunnel: [w924 w929 "*R27" "*R28"] -> w921
                                frame 0, Default {
                                n220 = Number To Hexadecimal String(1:i16 2 ("width (-)"), 2:"% LOW Sollwert 2") -> (0:w925:string)
                                n221 = Concatenate Strings("*W27", w925) -> (w924:string)
                                }
                                frame 1 {
                                n222 = Number To Hexadecimal String(1:i16 2 ("width (-)"), 2:"% High Sollwert 2") -> (0:w930:string)
                                n223 = Concatenate Strings("*W28", w930) -> (w929:string)
                                }
                                frame 2 {
                                }
                                frame 3 {
                                }
                              }
                            }
                            frame #1 {
                              n224 = Unbundle(w934) -> ("VISA resource name out"=w942:refnum<visa-resource-name>, "error out"=w940:errorcluster, "Delay (ms) 2"=w941:u32, "Write/\nRead \n\n2"=w939:bool)
                              n225 = call "I3252_Comm_Interface.vi"("VISA resource name in"=w942, "error in"=w940, "Delay (ms)"=w941, "Write"=w939, "String to Write"=w935, "Read"=w939) -> ("VISA resource name out"=w938:refnum<visa-resource-name>, "error out"=w937:errorcluster, "Read String"=w936:string)  [unwired: 2 in]
                            }
                            frame #2 {
                              n226 = case shown="3" w943 {
                                tunnel: w944 -> [_ w948 w952]
                                frame 0, Default {
                                }
                                frame 2 {
                                n227 = String Subset(string=w948, offset (0)=3) -> (substring=w946:string)  [unwired: 1 in]
                                n228 = Hexadecimal String To Number(string=w946) -> (number=→"% LOW Istwert 2":u32)  [unwired: 2 in, 1 out]
                                }
                                frame 3 {
                                n229 = String Subset(string=w952, offset (0)=3) -> (substring=w950:string)  [unwired: 1 in]
                                n230 = Hexadecimal String To Number(string=w950) -> (number=→"% HIGH Istwert 2":u32)  [unwired: 2 in, 1 out]
                                }
                              }
                            }
                          }
                        }
                      }
                      frame #2 {
                        n231 = property on="Write LOW/HI 2" class="Bool"("Blinking"=FALSE) -> ()  [unwired: 2 in, 2 out]
                      }
                    }
                    n232 = Not(x="Write LOW/HI 2") -> (.not. x?=w907:bool)
                    n233 = Unbundle(w905) -> ("VISA resource name out"=w904:refnum<visa-resource-name>, "error out"=w903:errorcluster)  [unwired: 2 out]
                  }
                  event "Set PID": Value Change {
                    n234 = event-data() -> ()  [unwired: 1 in, 1 out]
                    n235 = stacked-sequence {
                      tunnel: w959 -> [_ w966 _]
                      tunnel: [_ w965 _] -> w958
                      tunnel: [_ w964 _] -> w957
                      frame #0 {
                        n236 = property on="Set PID" class="Bool"("Blinking"=TRUE) -> ()  [unwired: 2 in, 2 out]
                        n237 = property on="ON" class="Bool (strict)"("Blinking"=FALSE) -> ()  [unwired: 2 in, 2 out]
                      }
                      frame #1 {
                        n238 = for {
                          N: 6 -> [_]
                          tunnel: w966 -> [w970]
                          tunnel: [w969] -> w965
                          tunnel: [w968] -> w964
                          i -> [w972]
                          n239 = flat-sequence {
                            tunnel: w972 -> [w974]
                            tunnel: [w975] -> w971
                            tunnel: w971 -> [w1016]
                            tunnel: [w1012] -> w973
                            tunnel: w970 -> [w1015]
                            tunnel: [w1014] -> w968
                            tunnel: [w1013] -> w969
                            tunnel: w973 -> [w1022]
                            tunnel: w972 -> [w1021]
                            frame #0 {
                              n240 = case shown="2" w974 {
                                tunnel: [w982 w990 w998 w1000 w1004 w1008] -> w975
                                frame 0, Default {
                                n241 = local read "RAM"() -> (w976:bool)
                                n242 = Number To Hexadecimal String(1:i16 4 ("width (-)"), 2:"P (PB1) Sollwert") -> (0:w983:string)
                                n243 = Select(t="*P17", s=w976, f="*W17") -> (s? t:f=w977:string)
                                n244 = Concatenate Strings(w977, w983) -> (w982:string)
                                }
                                frame 1 {
                                n245 = local read "RAM"() -> (w984:bool)
                                n246 = Number To Hexadecimal String(1:i16 4 ("width (-)"), 2:"I ( Reset1) Sollwert") -> (0:w991:string)
                                n247 = Select(t="*P18", s=w984, f="*W18") -> (s? t:f=w986:string)
                                n248 = Concatenate Strings(w986, w991) -> (w990:string)
                                }
                                frame 2 {
                                n249 = local read "RAM"() -> (w993:bool)
                                n250 = Number To Hexadecimal String(1:i16 4 ("width (-)"), 2:"D (Rate) Sollwert") -> (0:w999:string)
                                n251 = Select(t="*P19", s=w993, f="*W19") -> (s? t:f=w994:string)
                                n252 = Concatenate Strings(w994, w999) -> (w998:string)
                                }
                                frame 3 {
                                n253 = local read "RAM"() -> (w1003:bool)
                                n254 = Select(t="*G17", s=w1003, f="*R17") -> (s? t:f=w1000:string)
                                }
                                frame 4 {
                                n255 = local read "RAM"() -> (w1007:bool)
                                n256 = Select(t="*G18", s=w1007, f="*R18") -> (s? t:f=w1004:string)
                                }
                                frame 5 {
                                n257 = local read "RAM"() -> (w1011:bool)
                                n258 = Select(t="*G19", s=w1011, f="*R19") -> (s? t:f=w1008:string)
                                }
                              }
                            }
                            frame #1 {
                              n259 = Unbundle(w1015) -> ("VISA resource name out"=w1020:refnum<visa-resource-name>, "error out"=w1018:errorcluster, "Delay (ms)"=w1019:u32, "Write/\nRead"=w1017:bool)
                              n260 = call "I3252_Comm_Interface.vi"("VISA resource name in"=w1020, "error in"=w1018, "Delay (ms)"=w1019, "Write"=w1017, "String to Write"=w1016, "Read"=w1017) -> ("VISA resource name out"=w1013:refnum<visa-resource-name>, "error out"=w1014:errorcluster, "Read String"=w1012:string)  [unwired: 2 in]
                            }
                            frame #2 {
                              n261 = case shown="4" w1021 {
                                tunnel: w1022 -> [_ w1026 w1030 w1034]
                                frame 0, Default {
                                }
                                frame 3 {
                                n262 = String Subset(string=w1026, offset (0)=3) -> (substring=w1024:string)  [unwired: 1 in]
                                n263 = Hexadecimal String To Number(string=w1024) -> (number=→"P (PB1) Istwert":u32)  [unwired: 2 in, 1 out]
                                }
                                frame 4 {
                                n264 = String Subset(string=w1030, offset (0)=3) -> (substring=w1028:string)  [unwired: 1 in]
                                n265 = Hexadecimal String To Number(string=w1028) -> (number=→"I ( Reset1) Istwert":u32)  [unwired: 2 in, 1 out]
                                }
                                frame 5 {
                                n266 = String Subset(string=w1034, offset (0)=3) -> (substring=w1032:string)  [unwired: 1 in]
                                n267 = Hexadecimal String To Number(string=w1032) -> (number=→"D (Rate) IstWert":u32)  [unwired: 2 in, 1 out]
                                }
                              }
                            }
                          }
                        }
                      }
                      frame #2 {
                        n268 = property on="Set PID" class="Bool"("Blinking"=FALSE) -> ()  [unwired: 2 in, 2 out]
                      }
                    }
                    n269 = Not(x="Set PID") -> (.not. x?=w961:bool)
                    n270 = Unbundle(w956) -> ("VISA resource name out"=w955:refnum<visa-resource-name>, "error out"=w954:errorcluster)  [unwired: 2 out]
                  }
                  event "Set PID 2": Value Change {
                    n271 = event-data() -> ()  [unwired: 1 in, 1 out]
                    n272 = stacked-sequence {
                      tunnel: w1036 -> [_ w1048 _]
                      tunnel: [_ w1047 _] -> w1038
                      tunnel: [_ w1046 _] -> w1037
                      frame #0 {
                        n273 = property on="Set PID 2" class="Bool"("Blinking"=TRUE) -> ()  [unwired: 2 in, 2 out]
                        n274 = property on="ON 2" class="Bool (strict)"("Blinking"=FALSE) -> ()  [unwired: 2 in, 2 out]
                      }
                      frame #1 {
                        n275 = for {
                          N: 6 -> [_]
                          tunnel: w1048 -> [w1052]
                          tunnel: [w1051] -> w1047
                          tunnel: [w1050] -> w1046
                          i -> [w1054]
                          n276 = flat-sequence {
                            tunnel: w1054 -> [w1056]
                            tunnel: [w1057] -> w1053
                            tunnel: w1053 -> [w1098]
                            tunnel: [w1094] -> w1055
                            tunnel: w1052 -> [w1097]
                            tunnel: [w1096] -> w1050
                            tunnel: [w1095] -> w1051
                            tunnel: w1055 -> [w1104]
                            tunnel: w1054 -> [w1103]
                            frame #0 {
                              n277 = case shown="0, Default" w1056 {
                                tunnel: [w1064 w1072 w1080 w1082 w1086 w1090] -> w1057
                                frame 0, Default {
                                n278 = local read "RAM 2"() -> (w1059:bool)
                                n279 = Number To Hexadecimal String(1:i16 4 ("width (-)"), 2:"P (PB1) Sollwert 2") -> (0:w1065:string)
                                n280 = Select(t="*P17", s=w1059, f="*W17") -> (s? t:f=w1060:string)
                                n281 = Concatenate Strings(w1060, w1065) -> (w1064:string)
                                }
                                frame 1 {
                                n282 = local read "RAM 2"() -> (w1067:bool)
                                n283 = Number To Hexadecimal String(1:i16 4 ("width (-)"), 2:"I ( Reset1) Sollwert 2") -> (0:w1073:string)
                                n284 = Select(t="*P18", s=w1067, f="*W18") -> (s? t:f=w1068:string)
                                n285 = Concatenate Strings(w1068, w1073) -> (w1072:string)
                                }
                                frame 2 {
                                n286 = local read "RAM 2"() -> (w1075:bool)
                                n287 = Number To Hexadecimal String(1:i16 4 ("width (-)"), 2:"D (Rate) Sollwert 2") -> (0:w1081:string)
                                n288 = Select(t="*P19", s=w1075, f="*W19") -> (s? t:f=w1076:string)
                                n289 = Concatenate Strings(w1076, w1081) -> (w1080:string)
                                }
                                frame 3 {
                                n290 = local read "RAM"() -> (w1085:bool)
                                n291 = Select(t="*G17", s=w1085, f="*R17") -> (s? t:f=w1082:string)
                                }
                                frame 4 {
                                n292 = local read "RAM"() -> (w1089:bool)
                                n293 = Select(t="*G18", s=w1089, f="*R18") -> (s? t:f=w1086:string)
                                }
                                frame 5 {
                                n294 = local read "RAM"() -> (w1093:bool)
                                n295 = Select(t="*G19", s=w1093, f="*R19") -> (s? t:f=w1090:string)
                                }
                              }
                            }
                            frame #1 {
                              n296 = Unbundle(w1097) -> ("VISA resource name out"=w1102:refnum<visa-resource-name>, "error out"=w1100:errorcluster, "Delay (ms) 2"=w1101:u32, "Write/\nRead \n\n2"=w1099:bool)
                              n297 = call "I3252_Comm_Interface.vi"("VISA resource name in"=w1102, "error in"=w1100, "Delay (ms)"=w1101, "Write"=w1099, "String to Write"=w1098, "Read"=w1099) -> ("VISA resource name out"=w1095:refnum<visa-resource-name>, "error out"=w1096:errorcluster, "Read String"=w1094:string)  [unwired: 2 in]
                            }
                            frame #2 {
                              n298 = case shown="0, Default" w1103 {
                                tunnel: w1104 -> [_ w1108 w1112 w1116]
                                frame 0, Default {
                                }
                                frame 3 {
                                n299 = String Subset(string=w1108, offset (0)=3) -> (substring=w1106:string)  [unwired: 1 in]
                                n300 = Hexadecimal String To Number(string=w1106) -> (number=→"P (PB1) Istwert 2":u32)  [unwired: 2 in, 1 out]
                                }
                                frame 4 {
                                n301 = String Subset(string=w1112, offset (0)=3) -> (substring=w1110:string)  [unwired: 1 in]
                                n302 = Hexadecimal String To Number(string=w1110) -> (number=→"I ( Reset1) Istwert 2":u32)  [unwired: 2 in, 1 out]
                                }
                                frame 5 {
                                n303 = String Subset(string=w1116, offset (0)=3) -> (substring=w1114:string)  [unwired: 1 in]
                                n304 = Hexadecimal String To Number(string=w1114) -> (number=→"D (Rate) IstWert 2":u32)  [unwired: 2 in, 1 out]
                                }
                              }
                            }
                          }
                        }
                      }
                      frame #2 {
                        n305 = property on="Set PID 2" class="Bool"("Blinking"=FALSE) -> ()  [unwired: 2 in, 2 out]
                      }
                    }
                    n306 = Not(x="Set PID 2") -> (.not. x?=w1043:bool)
                    n307 = Unbundle(w1041) -> ("VISA resource name out"=w1040:refnum<visa-resource-name>, "error out"=w1039:errorcluster)  [unwired: 2 out]
                  }
                  event "Get Values": Value Change {
                    n308 = event-data() -> ()  [unwired: 1 in, 1 out]
                    n309 = stacked-sequence {
                      tunnel: w1123 -> [_ w1130 _]
                      tunnel: [_ w1129 _] -> w1122
                      tunnel: [_ w1128 _] -> w1121
                      frame #0 {
                        n310 = property on="Get Values" class="Bool"("Blinking"=TRUE) -> ()  [unwired: 2 in, 2 out]
                        n311 = property on="ON" class="Bool (strict)"("Blinking"=FALSE) -> ()  [unwired: 2 in, 2 out]
                      }
                      frame #1 {
                        n312 = for {
                          N: 6 -> [_]
                          tunnel: w1130 -> [w1134]
                          tunnel: [w1133] -> w1129
                          tunnel: [w1132] -> w1128
                          i -> [w1136]
                          n313 = flat-sequence {
                            tunnel: w1136 -> [w1138]
                            tunnel: [w1139] -> w1135
                            tunnel: w1135 -> [w1161]
                            tunnel: [w1162] -> w1137
                            tunnel: w1134 -> [w1160]
                            tunnel: [w1159] -> w1132
                            tunnel: [w1158] -> w1133
                            tunnel: w1137 -> [w1168]
                            tunnel: w1136 -> [w1167]
                            frame #0 {
                              n314 = case shown="0, Default" w1138 {
                                tunnel: [w1142 w1146 w1150 "*R27" "*R28" w1156] -> w1139
                                frame 0, Default {
                                n315 = local read "RAM"() -> (w1143:bool)
                                n316 = Select(t="*G17", s=w1143, f="*R17") -> (s? t:f=w1142:string)
                                }
                                frame 1 {
                                n317 = local read "RAM"() -> (w1147:bool)
                                n318 = Select(t="*G18", s=w1147, f="*R18") -> (s? t:f=w1146:string)
                                }
                                frame 2 {
                                n319 = local read "RAM"() -> (w1151:bool)
                                n320 = Select(t="*G19", s=w1151, f="*R19") -> (s? t:f=w1150:string)
                                }
                                frame 3 {
                                }
                                frame 4 {
                                }
                                frame 5 {
                                n321 = local read "RAM"() -> (w1157:bool)
                                n322 = Select(t="*G01", s=w1157, f="*R01") -> (s? t:f=w1156:string)
                                }
                              }
                            }
                            frame #1 {
                              n323 = Unbundle(w1160) -> ("VISA resource name out"=w1166:refnum<visa-resource-name>, "error out"=w1164:errorcluster, "Delay (ms)"=w1165:u32, "Write/\nRead"=w1163:bool)
                              n324 = call "I3252_Comm_Interface.vi"("VISA resource name in"=w1166, "error in"=w1164, "Delay (ms)"=w1165, "Write"=w1163, "String to Write"=w1161, "Read"=w1163) -> ("VISA resource name out"=w1158:refnum<visa-resource-name>, "error out"=w1159:errorcluster, "Read String"=w1162:string)  [unwired: 2 in]
                            }
                            frame #2 {
                              n325 = case shown="1" w1167 {
                                tunnel: w1168 -> [w1170 w1174 w1178 w1182 w1186 w1190]
                                frame 0, Default {
                                n326 = String Subset(string=w1170, offset (0)=3) -> (substring=w1171:string)  [unwired: 1 in]
                                n327 = Hexadecimal String To Number(string=w1171) -> (number=w1169:u32)  [unwired: 2 in, 1 out]
                                n328 = local write "P (PB1) Sollwert"(w1169) -> ()
                                n329 = local write "P (PB1) Istwert"(w1169) -> ()
                                }
                                frame 1 {
                                n330 = String Subset(string=w1174, offset (0)=3) -> (substring=w1175:string)  [unwired: 1 in]
                                n331 = Hexadecimal String To Number(string=w1175) -> (number=w1173:u32)  [unwired: 2 in, 1 out]
                                n332 = local write "I ( Reset1) Sollwert"(w1173) -> ()
                                n333 = local write "I ( Reset1) Istwert"(w1173) -> ()
                                }
                                frame 2 {
                                n334 = String Subset(string=w1178, offset (0)=3) -> (substring=w1179:string)  [unwired: 1 in]
                                n335 = Hexadecimal String To Number(string=w1179) -> (number=w1177:u32)  [unwired: 2 in, 1 out]
                                n336 = local write "D (Rate) Sollwert"(w1177) -> ()
                                n337 = local write "D (Rate) IstWert"(w1177) -> ()
                                }
                                frame 3 {
                                n338 = String Subset(string=w1182, offset (0)=3) -> (substring=w1183:string)  [unwired: 1 in]
                                n339 = Hexadecimal String To Number(string=w1183) -> (number=w1181:u32)  [unwired: 2 in, 1 out]
                                n340 = local write "% LOW Istwert"(w1181) -> ()
                                n341 = local write "% LOW Sollwert"(w1181) -> ()
                                }
                                frame 4 {
                                n342 = String Subset(string=w1186, offset (0)=3) -> (substring=w1187:string)  [unwired: 1 in]
                                n343 = Hexadecimal String To Number(string=w1187) -> (number=w1185:u32)  [unwired: 2 in, 1 out]
                                n344 = local write "% High Sollwert"(w1185) -> ()
                                n345 = local write "% HIGH Istwert"(w1185) -> ()
                                }
                                frame 5 {
                                n346 = call "I3252_Edit_Setpoint.vi"("Read String"=w1190) -> ("Setpoint is"=w1189:dbl)
                                n347 = local write "SP 1 is (°C)"(w1189) -> ()
                                }
                              }
                            }
                          }
                        }
                      }
                      frame #2 {
                        n348 = property on="Get Values" class="Bool"("Blinking"=FALSE) -> ()  [unwired: 2 in, 2 out]
                      }
                    }
                    n349 = Not(x="Get Values") -> (.not. x?=w1125:bool)
                    n350 = Unbundle(w1120) -> ("VISA resource name out"=w1119:refnum<visa-resource-name>, "error out"=w1118:errorcluster)  [unwired: 2 out]
                  }
                  event "Get Values 2": Value Change {
                    n351 = event-data() -> ()  [unwired: 1 in, 1 out]
                    n352 = stacked-sequence {
                      tunnel: w1194 -> [_ w1204 _]
                      tunnel: [_ w1203 _] -> w1193
                      tunnel: [_ w1202 _] -> w1192
                      frame #0 {
                        n353 = property on="Get Values 2" class="Bool"("Blinking"=TRUE) -> ()  [unwired: 2 in, 2 out]
                        n354 = property on="ON 2" class="Bool (strict)"("Blinking"=FALSE) -> ()  [unwired: 2 in, 2 out]
                      }
                      frame #1 {
                        n355 = for {
                          N: 6 -> [_]
                          tunnel: w1204 -> [w1208]
                          tunnel: [w1207] -> w1203
                          tunnel: [w1206] -> w1202
                          i -> [w1210]
                          n356 = flat-sequence {
                            tunnel: w1210 -> [w1212]
                            tunnel: [w1213] -> w1209
                            tunnel: w1209 -> [w1235]
                            tunnel: [w1236] -> w1211
                            tunnel: w1208 -> [w1234]
                            tunnel: [w1233] -> w1206
                            tunnel: [w1232] -> w1207
                            tunnel: w1211 -> [w1242]
                            tunnel: w1210 -> [w1241]
                            frame #0 {
                              n357 = case shown="1" w1212 {
                                tunnel: [w1216 w1220 w1224 "*R27" "*R28" w1230] -> w1213
                                frame 0, Default {
                                n358 = local read "RAM 2"() -> (w1217:bool)
                                n359 = Select(t="*G17", s=w1217, f="*R17") -> (s? t:f=w1216:string)
                                }
                                frame 1 {
                                n360 = local read "RAM 2"() -> (w1221:bool)
                                n361 = Select(t="*G18", s=w1221, f="*R18") -> (s? t:f=w1220:string)
                                }
                                frame 2 {
                                n362 = local read "RAM 2"() -> (w1225:bool)
                                n363 = Select(t="*G19", s=w1225, f="*R19") -> (s? t:f=w1224:string)
                                }
                                frame 3 {
                                }
                                frame 4 {
                                }
                                frame 5 {
                                n364 = local read "RAM 2"() -> (w1231:bool)
                                n365 = Select(t="*G01", s=w1231, f="*R01") -> (s? t:f=w1230:string)
                                }
                              }
                            }
                            frame #1 {
                              n366 = Unbundle(w1234) -> ("VISA resource name out"=w1240:refnum<visa-resource-name>, "error out"=w1238:errorcluster, "Delay (ms) 2"=w1239:u32, "Write/\nRead \n\n2"=w1237:bool)
                              n367 = call "I3252_Comm_Interface.vi"("VISA resource name in"=w1240, "error in"=w1238, "Delay (ms)"=w1239, "Write"=w1237, "String to Write"=w1235, "Read"=w1237) -> ("VISA resource name out"=w1232:refnum<visa-resource-name>, "error out"=w1233:errorcluster, "Read String"=w1236:string)  [unwired: 2 in]
                            }
                            frame #2 {
                              n368 = case shown="0, Default" w1241 {
                                tunnel: w1242 -> [w1244 w1248 w1252 w1256 w1260 w1264]
                                frame 0, Default {
                                n369 = String Subset(string=w1244, offset (0)=3) -> (substring=w1245:string)  [unwired: 1 in]
                                n370 = Hexadecimal String To Number(string=w1245) -> (number=w1243:u32)  [unwired: 2 in, 1 out]
                                n371 = local write "P (PB1) Sollwert 2"(w1243) -> ()
                                n372 = local write "P (PB1) Istwert 2"(w1243) -> ()
                                }
                                frame 1 {
                                n373 = String Subset(string=w1248, offset (0)=3) -> (substring=w1249:string)  [unwired: 1 in]
                                n374 = Hexadecimal String To Number(string=w1249) -> (number=w1247:u32)  [unwired: 2 in, 1 out]
                                n375 = local write "I ( Reset1) Sollwert 2"(w1247) -> ()
                                n376 = local write "I ( Reset1) Istwert 2"(w1247) -> ()
                                }
                                frame 2 {
                                n377 = String Subset(string=w1252, offset (0)=3) -> (substring=w1253:string)  [unwired: 1 in]
                                n378 = Hexadecimal String To Number(string=w1253) -> (number=w1251:u32)  [unwired: 2 in, 1 out]
                                n379 = local write "D (Rate) Sollwert 2"(w1251) -> ()
                                n380 = local write "D (Rate) IstWert 2"(w1251) -> ()
                                }
                                frame 3 {
                                n381 = String Subset(string=w1256, offset (0)=3) -> (substring=w1257:string)  [unwired: 1 in]
                                n382 = Hexadecimal String To Number(string=w1257) -> (number=w1255:u32)  [unwired: 2 in, 1 out]
                                n383 = local write "% LOW Istwert 2"(w1255) -> ()
                                n384 = local write "% LOW Sollwert 2"(w1255) -> ()
                                }
                                frame 4 {
                                n385 = String Subset(string=w1260, offset (0)=3) -> (substring=w1261:string)  [unwired: 1 in]
                                n386 = Hexadecimal String To Number(string=w1261) -> (number=w1259:u32)  [unwired: 2 in, 1 out]
                                n387 = local write "% High Sollwert 2"(w1259) -> ()
                                n388 = local write "% HIGH Istwert 2"(w1259) -> ()
                                }
                                frame 5 {
                                n389 = call "I3252_Edit_Setpoint.vi"("Read String"=w1264) -> ("Setpoint is"=w1263:dbl)
                                n390 = local write "SP 2 is (°C)"(w1263) -> ()
                                }
                              }
                            }
                          }
                        }
                      }
                      frame #2 {
                        n391 = property on="Get Values 2" class="Bool"("Blinking"=FALSE) -> ()  [unwired: 2 in, 2 out]
                      }
                    }
                    n392 = Not(x="Get Values 2") -> (.not. x?=w1199:bool)
                    n393 = Unbundle(w1195) -> ("VISA resource name out"=w1197:refnum<visa-resource-name>, "error out"=w1196:errorcluster)  [unwired: 2 out]
                  }
                  event "RAM": Value Change {
                    n394 = event-data() -> ()  [unwired: 1 in, 1 out]
                    n395 = stacked-sequence {
                      tunnel: w1271 -> [_ w1278 _]
                      tunnel: [_ w1277 _] -> w1270
                      tunnel: [_ w1276 _] -> w1269
                      frame #0 {
                        n396 = property on="RAM" class="Bool (strict)"("Blinking"=TRUE) -> ()  [unwired: 2 in, 2 out]
                        n397 = property on="ON" class="Bool (strict)"("Blinking"=FALSE) -> ()  [unwired: 2 in, 2 out]
                      }
                      frame #1 {
                        n398 = for {
                          N: 6 -> [_]
                          tunnel: w1278 -> [w1282]
                          tunnel: [w1281] -> w1277
                          tunnel: [w1280] -> w1276
                          i -> [w1284]
                          n399 = flat-sequence {
                            tunnel: w1284 -> [w1286]
                            tunnel: [w1287] -> w1283
                            tunnel: w1283 -> [w1306]
                            tunnel: [w1307] -> w1285
                            tunnel: w1282 -> [w1310]
                            tunnel: [w1309] -> w1280
                            tunnel: [w1308] -> w1281
                            tunnel: w1285 -> [w1316]
                            tunnel: w1284 -> [w1315]
                            frame #0 {
                              n400 = case shown="3" w1286 {
                                tunnel: [w1290 w1294 w1298 "*R27" "*R28" w1304] -> w1287
                                frame 0, Default {
                                n401 = local read "RAM"() -> (w1291:bool)
                                n402 = Select(t="*G17", s=w1291, f="*R17") -> (s? t:f=w1290:string)
                                }
                                frame 1 {
                                n403 = local read "RAM"() -> (w1295:bool)
                                n404 = Select(t="*G18", s=w1295, f="*R18") -> (s? t:f=w1294:string)
                                }
                                frame 2 {
                                n405 = local read "RAM"() -> (w1299:bool)
                                n406 = Select(t="*G19", s=w1299, f="*R19") -> (s? t:f=w1298:string)
                                }
                                frame 3 {
                                }
                                frame 4 {
                                }
                                frame 5 {
                                n407 = local read "RAM"() -> (w1305:bool)
                                n408 = Select(t="*G01", s=w1305, f="*R01") -> (s? t:f=w1304:string)
                                }
                              }
                            }
                            frame #1 {
                              n409 = Unbundle(w1310) -> ("VISA resource name out"=w1314:refnum<visa-resource-name>, "error out"=w1312:errorcluster, "Delay (ms)"=w1313:u32, "Write/\nRead"=w1311:bool)
                              n410 = call "I3252_Comm_Interface.vi"("VISA resource name in"=w1314, "error in"=w1312, "Delay (ms)"=w1313, "Write"=w1311, "String to Write"=w1306, "Read"=w1311) -> ("VISA resource name out"=w1308:refnum<visa-resource-name>, "error out"=w1309:errorcluster, "Read String"=w1307:string)  [unwired: 2 in]
                            }
                            frame #2 {
                              n411 = case shown="5" w1315 {
                                tunnel: w1316 -> [w1318 w1322 w1326 w1330 w1334 w1338]
                                frame 0, Default {
                                n412 = String Subset(string=w1318, offset (0)=3) -> (substring=w1319:string)  [unwired: 1 in]
                                n413 = Hexadecimal String To Number(string=w1319) -> (number=w1317:u32)  [unwired: 2 in, 1 out]
                                n414 = local write "P (PB1) Sollwert"(w1317) -> ()
                                n415 = local write "P (PB1) Istwert"(w1317) -> ()
                                }
                                frame 1 {
                                n416 = String Subset(string=w1322, offset (0)=3) -> (substring=w1323:string)  [unwired: 1 in]
                                n417 = Hexadecimal String To Number(string=w1323) -> (number=w1321:u32)  [unwired: 2 in, 1 out]
                                n418 = local write "I ( Reset1) Sollwert"(w1321) -> ()
                                n419 = local write "I ( Reset1) Istwert"(w1321) -> ()
                                }
                                frame 2 {
                                n420 = String Subset(string=w1326, offset (0)=3) -> (substring=w1327:string)  [unwired: 1 in]
                                n421 = Hexadecimal String To Number(string=w1327) -> (number=w1325:u32)  [unwired: 2 in, 1 out]
                                n422 = local write "D (Rate) IstWert"(w1325) -> ()
                                n423 = local write "D (Rate) Sollwert"(w1325) -> ()
                                }
                                frame 3 {
                                n424 = String Subset(string=w1330, offset (0)=3) -> (substring=w1331:string)  [unwired: 1 in]
                                n425 = Hexadecimal String To Number(string=w1331) -> (number=w1329:u32)  [unwired: 2 in, 1 out]
                                n426 = local write "% LOW Istwert"(w1329) -> ()
                                n427 = local write "% LOW Sollwert"(w1329) -> ()
                                }
                                frame 4 {
                                n428 = String Subset(string=w1334, offset (0)=3) -> (substring=w1335:string)  [unwired: 1 in]
                                n429 = Hexadecimal String To Number(string=w1335) -> (number=w1333:u32)  [unwired: 2 in, 1 out]
                                n430 = local write "% HIGH Istwert"(w1333) -> ()
                                n431 = local write "% High Sollwert"(w1333) -> ()
                                }
                                frame 5 {
                                n432 = call "I3252_Edit_Setpoint.vi"("Read String"=w1338) -> ("Setpoint is"=w1337:dbl)
                                n433 = local write "SP 1 is (°C)"(w1337) -> ()
                                }
                              }
                            }
                          }
                        }
                      }
                      frame #2 {
                        n434 = property on="RAM" class="Bool (strict)"("Blinking"=FALSE) -> ()  [unwired: 2 in, 2 out]
                      }
                    }
                    n435 = Not(x="RAM") -> (.not. x?=w1273:bool)
                    n436 = Unbundle(w1268) -> ("VISA resource name out"=w1267:refnum<visa-resource-name>, "error out"=w1266:errorcluster)  [unwired: 2 out]
                  }
                  event "RAM 2": Value Change {
                    n437 = event-data() -> ()  [unwired: 1 in, 1 out]
                    n438 = stacked-sequence {
                      tunnel: w1342 -> [_ w1352 _]
                      tunnel: [_ w1351 _] -> w1341
                      tunnel: [_ w1350 _] -> w1340
                      frame #0 {
                        n439 = property on="RAM 2" class="Bool (strict)"("Blinking"=TRUE) -> ()  [unwired: 2 in, 2 out]
                        n440 = property on="ON 2" class="Bool (strict)"("Blinking"=FALSE) -> ()  [unwired: 2 in, 2 out]
                      }
                      frame #1 {
                        n441 = for {
                          N: 6 -> [_]
                          tunnel: w1352 -> [w1356]
                          tunnel: [w1355] -> w1351
                          tunnel: [w1354] -> w1350
                          i -> [w1358]
                          n442 = flat-sequence {
                            tunnel: w1358 -> [w1360]
                            tunnel: [w1361] -> w1357
                            tunnel: w1357 -> [w1380]
                            tunnel: [w1381] -> w1359
                            tunnel: w1356 -> [w1384]
                            tunnel: [w1383] -> w1354
                            tunnel: [w1382] -> w1355
                            tunnel: w1359 -> [w1390]
                            tunnel: w1358 -> [w1389]
                            frame #0 {
                              n443 = case shown="5" w1360 {
                                tunnel: [w1364 w1368 w1372 "*R27" "*R28" w1378] -> w1361
                                frame 0, Default {
                                n444 = local read "RAM 2"() -> (w1365:bool)
                                n445 = Select(t="*G17", s=w1365, f="*R17") -> (s? t:f=w1364:string)
                                }
                                frame 1 {
                                n446 = local read "RAM 2"() -> (w1369:bool)
                                n447 = Select(t="*G18", s=w1369, f="*R18") -> (s? t:f=w1368:string)
                                }
                                frame 2 {
                                n448 = local read "RAM 2"() -> (w1373:bool)
                                n449 = Select(t="*G19", s=w1373, f="*R19") -> (s? t:f=w1372:string)
                                }
                                frame 3 {
                                }
                                frame 4 {
                                }
                                frame 5 {
                                n450 = local read "RAM 2"() -> (w1379:bool)
                                n451 = Select(t="*G01", s=w1379, f="*R01") -> (s? t:f=w1378:string)
                                }
                              }
                            }
                            frame #1 {
                              n452 = Unbundle(w1384) -> ("VISA resource name out"=w1388:refnum<visa-resource-name>, "error out"=w1386:errorcluster, "Delay (ms) 2"=w1387:u32, "Write/\nRead \n\n2"=w1385:bool)
                              n453 = call "I3252_Comm_Interface.vi"("VISA resource name in"=w1388, "error in"=w1386, "Delay (ms)"=w1387, "Write"=w1385, "String to Write"=w1380, "Read"=w1385) -> ("VISA resource name out"=w1382:refnum<visa-resource-name>, "error out"=w1383:errorcluster, "Read String"=w1381:string)  [unwired: 2 in]
                            }
                            frame #2 {
                              n454 = case shown="0, Default" w1389 {
                                tunnel: w1390 -> [w1392 w1396 w1400 w1404 w1408 w1412]
                                frame 0, Default {
                                n455 = String Subset(string=w1392, offset (0)=3) -> (substring=w1393:string)  [unwired: 1 in]
                                n456 = Hexadecimal String To Number(string=w1393) -> (number=w1391:u32)  [unwired: 2 in, 1 out]
                                n457 = local write "P (PB1) Sollwert 2"(w1391) -> ()
                                n458 = local write "P (PB1) Istwert 2"(w1391) -> ()
                                }
                                frame 1 {
                                n459 = String Subset(string=w1396, offset (0)=3) -> (substring=w1397:string)  [unwired: 1 in]
                                n460 = Hexadecimal String To Number(string=w1397) -> (number=w1395:u32)  [unwired: 2 in, 1 out]
                                n461 = local write "I ( Reset1) Sollwert 2"(w1395) -> ()
                                n462 = local write "I ( Reset1) Istwert 2"(w1395) -> ()
                                }
                                frame 2 {
                                n463 = String Subset(string=w1400, offset (0)=3) -> (substring=w1401:string)  [unwired: 1 in]
                                n464 = Hexadecimal String To Number(string=w1401) -> (number=w1399:u32)  [unwired: 2 in, 1 out]
                                n465 = local write "D (Rate) IstWert 2"(w1399) -> ()
                                n466 = local write "D (Rate) Sollwert 2"(w1399) -> ()
                                }
                                frame 3 {
                                n467 = String Subset(string=w1404, offset (0)=3) -> (substring=w1405:string)  [unwired: 1 in]
                                n468 = Hexadecimal String To Number(string=w1405) -> (number=w1403:u32)  [unwired: 2 in, 1 out]
                                n469 = local write "% LOW Istwert 2"(w1403) -> ()
                                n470 = local write "% LOW Sollwert 2"(w1403) -> ()
                                }
                                frame 4 {
                                n471 = String Subset(string=w1408, offset (0)=3) -> (substring=w1409:string)  [unwired: 1 in]
                                n472 = Hexadecimal String To Number(string=w1409) -> (number=w1407:u32)  [unwired: 2 in, 1 out]
                                n473 = local write "% HIGH Istwert 2"(w1407) -> ()
                                n474 = local write "% High Sollwert 2"(w1407) -> ()
                                }
                                frame 5 {
                                n475 = call "I3252_Edit_Setpoint.vi"("Read String"=w1412) -> ("Setpoint is"=w1411:dbl)
                                n476 = local write "SP 2 is (°C)"(w1411) -> ()
                                }
                              }
                            }
                          }
                        }
                      }
                      frame #2 {
                        n477 = property on="RAM 2" class="Bool (strict)"("Blinking"=FALSE) -> ()  [unwired: 2 in, 2 out]
                      }
                    }
                    n478 = Not(x="RAM 2") -> (.not. x?=w1347:bool)
                    n479 = Unbundle(w1345) -> ("VISA resource name out"=w1344:refnum<visa-resource-name>, "error out"=w1343:errorcluster)  [unwired: 2 out]
                  }
                  event "Set Gauge to Zero": Value Change {
                    n480 = event-data() -> ()  [unwired: 1 in, 1 out]
                    n481 = flat-sequence {
                      tunnel: w1421 -> [w1426]
                      tunnel: [w1426] -> w1420
                      tunnel: w1420 -> [w1428]
                      tunnel: [w1432] -> w1419
                      tunnel: [w1431] -> w1418
                      tunnel: [w1428] -> w1417
                      tunnel: w1419 -> [w1438]
                      tunnel: w1418 -> [w1437]
                      tunnel: w1417 -> [w1433]
                      frame #0 {
                        n482 = property on="Set Gauge to Zero" class="Bool"("Blinking"=TRUE) -> ()  [unwired: 2 in, 2 out]
                      }
                      frame #1 {
                        w1429 = 0 items=["sensor 1", "sensor 2", "test"] ("Sensor Nr.:")
                        n483 = call "DUAL GAUGE-Get Pressure,Status.vi"("Sensor Nr.:"=w1429, "Referenz in"=w1428) -> ("Pressure"=w1432:dbl)  [unwired: 6 in, 3 out]
                        n484 = call "DUAL GAUGE-Offset display.vi"("W/R"=FALSE, "Referenz in"=w1428) -> ("Sensor 1 Get"=w1431:dbl)  [unwired: 6 in, 3 out]
                      }
                      frame #2 {
                        n485 = Add(x=w1438, y=w1437) -> (x+y=w1434:dbl)
                        n486 = call "DUAL GAUGE-Offset display.vi"("W/R"=TRUE, "Sensor 1 Set"=w1434, "Referenz in"=w1433) -> ("Sensor 1 Get"=→"Current Offset (mbar)":dbl)  [unwired: 5 in, 3 out]
                      }
                      frame #3 {
                        n487 = property on="Set Gauge to Zero" class="Bool"("Blinking"=TRUE) -> ()  [unwired: 2 in, 2 out]
                      }
                    }
                    n488 = Unbundle(w1425) -> ("VISA resource name out"=w1424:refnum<visa-resource-name>, "error out"=w1423:errorcluster)  [unwired: 2 out]
                    n489 = Unbundle(w1416) -> ("VISA resource name out"=w1415:refnum<visa-resource-name>, "error out"=w1414:errorcluster)  [unwired: 2 out]
                  }
                  event "Write to File": Value Change {
                    n490 = event-data() -> ("NewVal"=w1447:bool)  [unwired: 1 in]
                    n491 = Unbundle(w1450) -> ("VISA resource name out"=w1449:refnum<visa-resource-name>, "error out"=w1448:errorcluster)  [unwired: 2 out]
                    n492 = local read "File Path"() -> (w1443:path)
                    n493 = case shown="False" w1447 {
                      tunnel: w1443 -> [_ w1455]
                      tunnel: "User" -> [_ w1454]
                      tunnel: "Sample" -> [_ w1453]
                      tunnel: [path "" ("File Path") w1452] -> w1444
                      frame False {
                      }
                      frame True {
                        n494 = call "Header.vi"("Sample"=w1453, "User"=w1454, "File Path"=w1455) -> ("File Path"=w1452:path)
                      }
                    }
                    n495 = local write "File Path"(w1444) -> ()
                    n496 = Unbundle(w1442) -> ("VISA resource name out"=w1441:refnum<visa-resource-name>, "error out"=w1440:errorcluster)  [unwired: 2 out]
                  }
                }
              }
              n497 = Bundle(cluster=w425, "VISA resource name out"=w424, "error out"=w423) -> (w422:T7)  [unwired: 2 in]
              n498 = Bundle(cluster=w401, "VISA resource name out"=w403, "error out"=w402) -> (w400:T8)  [unwired: 2 in]
            }
            frame #2 {
            }
            frame #3 {
              (unwired) "Daniel Schuster (geb. 20.03.1988)"
              n499 = node-c288(w1517) -> (w1526:T3)  [unwired: 2 in]
              n500 = node-c288(w1532) -> (w1535:T3)  [unwired: 2 in]
              n501 = node-c288(w1522) -> (w1524:T3)  [unwired: 2 in]
              n502 = node-c288(w1531) -> (w1539:T3)  [unwired: 2 in]
              n503 = timed-sequence {
                timing: w1526 -> [_]
                timing-out: [_] -> w1525
                tunnel: w1501 -> [w1611]
                tunnel: w1500 -> [w1607]
                tunnel: [w1610] -> w1493
                tunnel: w1492 -> [w1609]
                tunnel: w1491 -> [w1608]
                tunnel: [w1606] -> w1490
                tunnel: [w1605] -> w1489
                tunnel: [w1604] -> w1487
                n504 = timed-flat-sequence {
                  tunnel: w1611 -> [w1620]
                  tunnel: [w1619] -> w1610
                  tunnel: w1609 -> [w1618]
                  tunnel: w1608 -> [w1617]
                  tunnel: w1607 -> [w1616]
                  tunnel: [w1614] -> w1606
                  tunnel: [w1613] -> w1605
                  tunnel: [w1612] -> w1604
                  n505 = node-c288() -> ()  [unwired: 1 in, 1 out]
                  n506 = case shown="True" "ON (TPG 2)" {
                    tunnel: w1616 -> [w1625 w1631]
                    tunnel: w1617 -> [w1624 w1630]
                    tunnel: [w1623 w1629] -> w1613
                    tunnel: [w1622 w1628] -> w1612
                    frame False {
                      w1626 = 0.0 ("Pressure")
                      n507 = property on="ON (TPG 2)" class="Bool (strict)"("Blinking"=FALSE) -> ()  [unwired: 2 in, 2 out]
                      n508 = Bundle("Pressure"=w1626, "Pressure"=w1626) -> (w1623:cluster{"Pressure":dbl, "Pressure":dbl})  [unwired: 1 in]
                      n509 = Bundle("TPG 2 COM"=w1625, "error out"=w1624) -> (w1622:T9)  [unwired: 1 in]
                    }
                    frame True {
                      n510 = stacked-sequence {
                        tunnel: w1631 -> [_ w1644]
                        tunnel: [_ w1640] -> w1629
                        tunnel: [_ w1636] -> w1628
                        tunnel: w1630 -> [_ w1633]
                        frame #0 {
                          n511 = property on="ON (TPG 2)" class="Bool (strict)"("Blinking"=TRUE) -> ()  [unwired: 2 in, 2 out]
                        }
                        frame #1 {
                          n512 = call "PresureGetSubVI.vi"("COM in"=w1644, "Fehler (Eingang)"=w1633) -> ("Status Gauge#1"=→"Status Gauge 2#1":i32, "Status Gauge#2"=→"Status Gauge 2#2":i32, "COM out"=w1637:refnum<visa-resource-name>, "Pressure Gauge#1"=w1638:dbl, "Pressure Gauge#2"=w1641:dbl, "Cluster (Ausgang)"=w1634:errorcluster)  [unwired: 12 in]
                          "Pressure Gauge 2#1" <- w1638
                          "Pressure Gauge 2#2" <- w1641
                          n513 = Bundle("COM out"=w1637, "Cluster (Ausgang)"=w1634) -> (w1636:T10)  [unwired: 1 in]
                          n514 = Unbundle(w1634) -> ("status"=w1635:bool, "code"=w1639:i32)  [unwired: 1 out]
                          n515 = Bundle("status"=w1635, "code"=w1639) -> ()  [unwired: 1 in, 1 out]
                          n516 = Bundle("Pressure Gauge#1"=w1638, "Pressure Gauge#2"=w1641) -> (w1640:T11)  [unwired: 1 in]
                        }
                      }
                    }
                  }
                  n517 = case shown="True" "ON (TPG 1)" {
                    tunnel: w1620 -> [w1648 w1654]
                    tunnel: [w1647 w1653] -> w1619
                    tunnel: w1618 -> [w1646 w1652]
                    tunnel: [w1645 w1651] -> w1614
                    frame False {
                      w1649 = 0.0 ("Pressure")
                      n518 = property on="ON (TPG 1)" class="Bool (strict)"("Blinking"=FALSE) -> ()  [unwired: 2 in, 2 out]
                      n519 = Bundle("Pressure"=w1649, "Pressure"=w1649) -> (w1645:cluster{"Pressure":dbl, "Pressure":dbl})  [unwired: 1 in]
                      n520 = Bundle("TPG 1 COM"=w1648, "error out"=w1646) -> (w1647:T12)  [unwired: 1 in]
                    }
                    frame True {
                      n521 = stacked-sequence {
                        tunnel: w1654 -> [_ w1667]
                        tunnel: [_ w1660] -> w1653
                        tunnel: w1652 -> [_ w1657]
                        tunnel: [_ w1656] -> w1651
                        frame #0 {
                          n522 = property on="ON (TPG 1)" class="Bool (strict)"("Blinking"=TRUE) -> ()  [unwired: 2 in, 2 out]
                        }
                        frame #1 {
                          n523 = call "PresureGetSubVI.vi"("COM in"=w1667, "Fehler (Eingang)"=w1657) -> ("Status Gauge#1"=→"Status Gauge 1#1":i32, "Status Gauge#2"=→"Status Gauge 1#2":i32, "COM out"=w1661:refnum<visa-resource-name>, "Pressure Gauge#1"=w1662:dbl, "Pressure Gauge#2"=w1664:dbl, "Cluster (Ausgang)"=w1658:errorcluster)  [unwired: 12 in]
                          "Pressure Gauge 1#1" <- w1662
                          "Pressure Gauge 1#2" <- w1664
                          n524 = Bundle("COM out"=w1661, "Cluster (Ausgang)"=w1658) -> (w1660:T10)  [unwired: 1 in]
                          n525 = Unbundle(w1658) -> ("status"=w1659:bool, "code"=w1663:i32)  [unwired: 1 out]
                          n526 = Bundle("status"=w1659, "code"=w1663) -> ()  [unwired: 1 in, 1 out]
                          n527 = Bundle("Pressure Gauge#1"=w1662, "Pressure Gauge#2"=w1664) -> (w1656:T11)  [unwired: 1 in]
                        }
                      }
                    }
                  }
                  n528 = node-c288() -> ()  [unwired: 1 in, 1 out]
                }
              }
              n529 = timed-sequence {
                timing: w1535 -> [_]
                timing-out: [_] -> w1534
                tunnel: w1533 -> [w1677]
                tunnel: [w1676] -> w1528
                tunnel: [w1675] -> w1527
                tunnel: [w1674] -> w1514
                n530 = timed-flat-sequence {
                  tunnel: w1677 -> [w1681]
                  tunnel: [w1680] -> w1676
                  tunnel: [w1679] -> w1675
                  tunnel: [w1678] -> w1674
                  n531 = node-c288() -> ()  [unwired: 1 in, 1 out]
                  n532 = case shown="False" "ON" {
                    tunnel: w1681 -> [w1685 w1690]
                    tunnel: [w1684 w1689] -> w1680
                    tunnel: [w1683 w1688] -> w1679
                    tunnel: [_ w1687] -> w1678
                    frame False {
                      n533 = Unbundle(w1685) -> ("VISA resource name out"=w1684:refnum<visa-resource-name>, "error out"=w1683:errorcluster)  [unwired: 2 out]
                      n534 = property on="ON" class="Bool (strict)"("Blinking"=FALSE) -> ()  [unwired: 2 in, 2 out]
                    }
                    frame True {
                      n535 = stacked-sequence {
                        tunnel: w1690 -> [_ w1695]
                        tunnel: [_ w1694] -> w1689
                        tunnel: [_ w1693] -> w1688
                        tunnel: [_ w1692] -> w1687
                        frame #0 {
                          n536 = property on="ON" class="Bool (strict)"("Blinking"=TRUE) -> ()  [unwired: 2 in, 2 out]
                        }
                        frame #1 {
                          n537 = Unbundle(w1695) -> ("VISA resource name out"=w1699:refnum<visa-resource-name>, "error out"=w1697:errorcluster, "Delay (ms)"=w1698:u32, "Write/\nRead"=w1696:bool)
                          n538 = call "I3252_Comm_Interface.vi"("VISA resource name in"=w1699, "error in"=w1697, "Delay (ms)"=w1698, "Write"=w1696, "String to Write"="*V01", "Read"=w1696) -> ("VISA resource name out"=w1694:refnum<visa-resource-name>, "error out"=w1693:errorcluster, "Read String"=w1692:string)  [unwired: 2 in]
                        }
                      }
                    }
                  }
                  n539 = node-c288() -> ()  [unwired: 1 in, 1 out]
                }
              }
              n540 = timed-sequence {
                timing: w1524 -> [_]
                timing-out: [_] -> w1523
                tunnel: w1521 -> [w1573]
                tunnel: w1520 -> [w1572]
                tunnel: [w1571] -> w1518
                tunnel: [w1570] -> w1519
                tunnel: [w1569] -> w1515
                n541 = timed-flat-sequence {
                  tunnel: w1573 -> [w1578]
                  tunnel: w1572 -> [w1577]
                  tunnel: [w1576] -> w1571
                  tunnel: [w1575] -> w1570
                  tunnel: [w1574] -> w1569
                  n542 = node-c288() -> ()  [unwired: 1 in, 1 out]
                  n543 = case shown="False" "ON" {
                    tunnel: w1578 -> [w1582 w1588]
                    tunnel: w1577 -> [w1583 w1587]
                    tunnel: [w1582 w1586] -> w1576
                    tunnel: [w1583 w1585] -> w1575
                    tunnel: [0.0 ("Reading") w1584] -> w1574
                    frame False {
                      n544 = property on="ON" class="Bool (strict)"("Blinking"=FALSE) -> ()  [unwired: 2 in, 2 out]
                    }
                    frame True {
                      n545 = stacked-sequence {
                        tunnel: w1588 -> [_ w1595]
                        tunnel: w1587 -> [_ w1594]
                        tunnel: [_ w1593] -> w1586
                        tunnel: [_ w1592] -> w1585
                        tunnel: [_ w1590] -> w1584
                        frame #0 {
                          n546 = property on="ON" class="Bool (strict)"("Blinking"=TRUE) -> ()  [unwired: 2 in, 2 out]
                        }
                        frame #1 {
                          n547 = call "VC840_Read.vi"("error in (no error)"=w1594, "VISA resource name"=w1595) -> ("error out"=w1592:errorcluster, "Unit"=→"Unit 2":string, "Reading"=w1590:dbl, "VISA resource name out"=w1593:refnum<visa-resource-name>, "Status"=→"Status 2":T2, "Mode"=→"Mode 2":enum16{"?", "Diode", "Beep", "DC", "AC"})  [unwired: 4 out]
                          "Reading 2" <- w1590
                        }
                      }
                    }
                  }
                  n548 = node-c288() -> ()  [unwired: 1 in, 1 out]
                }
              }
              n549 = timed-sequence {
                timing: w1539 -> [_]
                timing-out: [_] -> w1538
                tunnel: w1537 -> [w1711]
                tunnel: w1536 -> [w1710]
                tunnel: [w1709] -> w1530
                tunnel: [w1708] -> w1529
                tunnel: [w1707] -> w1516
                n550 = timed-flat-sequence {
                  tunnel: w1711 -> [w1716]
                  tunnel: w1710 -> [w1715]
                  tunnel: [w1714] -> w1709
                  tunnel: [w1713] -> w1708
                  tunnel: [w1712] -> w1707
                  n551 = node-c288() -> ()  [unwired: 1 in, 1 out]
                  n552 = case shown="True" "ON" {
                    tunnel: w1716 -> [w1720 w1726]
                    tunnel: w1715 -> [w1721 w1725]
                    tunnel: [w1720 w1724] -> w1714
                    tunnel: [w1721 w1723] -> w1713
                    tunnel: [0.0 ("Reading") w1722] -> w1712
                    frame False {
                      n553 = property on="ON" class="Bool (strict)"("Blinking"=FALSE) -> ()  [unwired: 2 in, 2 out]
                    }
                    frame True {
                      n554 = stacked-sequence {
                        tunnel: w1726 -> [_ w1733]
                        tunnel: w1725 -> [_ w1732]
                        tunnel: [_ w1731] -> w1724
                        tunnel: [_ w1730] -> w1723
                        tunnel: [_ w1728] -> w1722
                        frame #0 {
                          n555 = property on="ON" class="Bool (strict)"("Blinking"=TRUE) -> ()  [unwired: 2 in, 2 out]
                        }
                        frame #1 {
                          n556 = call "VC840_Read.vi"("error in (no error)"=w1732, "VISA resource name"=w1733) -> ("error out"=w1730:errorcluster, "Unit"=→"Unit 1":string, "Reading"=w1728:dbl, "VISA resource name out"=w1731:refnum<visa-resource-name>, "Status"=→"Status 1":T2, "Mode"=→"Mode 1":enum16{"?", "Diode", "Beep", "DC", "AC"})  [unwired: 4 out]
                          "Reading 1" <- w1728
                        }
                      }
                    }
                  }
                  n557 = node-c288() -> ()  [unwired: 1 in, 1 out]
                }
              }
              n558 = Tick Count (ms)() -> (millisecond timer value=w1502:u32)
              n559 = Subtract(x=w1502, y=w1507) -> (x-y=w1506:u32)
              n560 = Divide(x=w1506, y=u32 1000) -> (x/y=w1504:dbl)
              n561 = node-c288(w1534) -> ()  [unwired: 1 out]
              n562 = node-c288(w1538) -> ()  [unwired: 1 out]
              n563 = node-c288(w1523) -> ()  [unwired: 1 out]
              n564 = node-c288() -> (w1485:T3)  [unwired: 3 in]
              n565 = To Double Precision Float(number=w1504) -> (double precision float=w1508:dbl)
              "current time (s)" <- w1508
              n566 = timed-sequence {
                timing: w1485 -> [_]
                timing-out: [_] -> w1484
                tunnel: w1483 -> [w1543]
                tunnel: [w1542] -> w1480
                tunnel: [w1541] -> w1479
                tunnel: [w1540] -> w1482
                n567 = timed-flat-sequence {
                  tunnel: w1543 -> [w1548]
                  tunnel: [w1547] -> w1542
                  tunnel: [w1546] -> w1541
                  tunnel: [w1545] -> w1540
                  n568 = node-c288() -> ()  [unwired: 1 in, 1 out]
                  n569 = case shown="True" "ON 2" {
                    tunnel: w1548 -> [w1551 w1555]
                    tunnel: [w1550 w1554] -> w1547
                    tunnel: [w1549 w1553] -> w1546
                    tunnel: [_ w1552] -> w1545
                    frame False {
                      (unwired) FALSE
                      n570 = Unbundle(w1551) -> ("VISA resource name out"=w1550:refnum<visa-resource-name>, "error out"=w1549:errorcluster)  [unwired: 2 out]
                    }
                    frame True {
                      n571 = stacked-sequence {
                        tunnel: w1555 -> [_ w1559]
                        tunnel: [_ w1558] -> w1554
                        tunnel: [_ w1557] -> w1553
                        tunnel: [_ w1556] -> w1552
                        frame #0 {
                          (unwired) TRUE
                        }
                        frame #1 {
                          n572 = Unbundle(w1559) -> ("VISA resource name out"=w1563:refnum<visa-resource-name>, "error out"=w1561:errorcluster, "Delay (ms) 2"=w1562:u32, "Write/\nRead \n\n2"=w1560:bool)
                          n573 = call "I3252_Comm_Interface.vi"("VISA resource name in"=w1563, "error in"=w1561, "Delay (ms)"=w1562, "Write"=w1560, "String to Write"="*V01", "Read"=w1560) -> ("VISA resource name out"=w1558:refnum<visa-resource-name>, "error out"=w1557:errorcluster, "Read String"=w1556:string)  [unwired: 2 in]
                        }
                      }
                    }
                  }
                  n574 = node-c288() -> ()  [unwired: 1 in, 1 out]
                }
              }
              n575 = node-c288(w1525) -> ()  [unwired: 1 out]
              n576 = Unbundle(w1489) -> ("Pressure Gauge#1"=w1488:dbl, "Pressure Gauge#2"=w1486:dbl)
              "Pressure OpenPort2" <- w1486
              "Pressure Pirani 2" <- w1488
              n577 = Unbundle(w1490) -> ("Pressure Gauge#1"=w1499:dbl, "Pressure Gauge#2"=w1494:dbl)
              "Pressure Baratron 2" <- w1499
              "Pressure FullRange 2" <- w1494
              n578 = node-c288(w1484) -> ()  [unwired: 1 out]
            }
            frame #4 {
              n579 = Build Array (concatenate)(w1759, w1763) -> (w1758:dbl[])
              n580 = Build Array (concatenate)(w1762, w1764) -> (w1757:dbl[])
              n581 = Build Array (concatenate)(w1760, w1751) -> (w1755:dbl[])
              n582 = Build Array (concatenate)(w1761, w1752) -> (w1756:dbl[])
              n583 = Greater?(x=w1783, y="Pressure Limit (mbar)") -> (0:w1786:bool)
              n584 = case shown="False" w1786 {
                frame False {
                  n585 = property on="Standby" class="Bool (strict)"("DisabledEnum"=T6."Enabled" ("Disabled")) -> ()  [unwired: 2 in, 2 out]
                }
                frame True {
                  n586 = property on="Standby" class="Bool (strict)"("Val(Sgnl)"=TRUE ("Standby"), "DisabledEnum"=T6."Disabled" ("Disabled")) -> ()  [unwired: 2 in, 2 out]
                }
              }
              n587 = call "Resistivity_Calculation.vi"("Reading 1 (V)"=w1776, "Constant"="4PP constant", "Thickness (nm)"="Thickness (nm)", "Reading 2 (A)"=w1784) -> ("Resivtivity (Ohm*cm)"=w1768:dbl, "Current"=w1769:dbl, "Voltage"=w1770:dbl)
              "Resistivity (Ohm*cm)" <- w1768
              "Voltage (V)" <- w1770
              "Current (A)" <- w1769
              n588 = call "I3252_Edit_Temperature.vi"("Temp. String"=w1785) -> ("Temp. (°C)"=w1779:dbl)
              "(°C)" <- w1779
              n589 = call "I3252_Edit_Temperature.vi"("Temp. String"=w1747) -> ("Temp. (°C)"=w1746:dbl)
              "(°C) 2" <- w1746
              n590 = Build Array (concatenate)(w1781, w1782) -> (w1778:dbl[])
              n591 = Build Array (concatenate)(w1780, w1779) -> (w1766:dbl[])
              n592 = Build Array (concatenate)(w1744, w1746) -> (w1745:dbl[])
              n593 = Build Array (concatenate)(w1777, w1770) -> (w1775:dbl[])
              n594 = Build Array (concatenate)(w1774, w1769) -> (w1772:dbl[])
              n595 = Build Array (concatenate)(w1773, w1768) -> (w1771:dbl[])
              n596 = Build Array(w1770, w1769, w1768) -> (w1767:dbl[])
            }
            frame #5 {
              n597 = Bundle(w1801, w1818) -> (→"CMR275 Baratron":cluster{dbl[], dbl[]})  [unwired: 1 in]
              n598 = Bundle(w1801, w1817) -> (→"PKR251 FullRange":cluster{dbl[], dbl[]})  [unwired: 1 in]
              n599 = Bundle(w1801, w1816) -> (→"Pirani (VVP1 Scroll)":cluster{dbl[], dbl[]})  [unwired: 1 in]
              n600 = Bundle(w1801, w1815) -> (→"Pressure OpenPort":cluster{dbl[], dbl[]})  [unwired: 1 in]
              n601 = Bundle(w1801, w1824) -> (→"Thermocouple (Sample holder 1)":cluster{dbl[], dbl[]})  [unwired: 1 in]
              n602 = Bundle(w1801, w1826) -> (→"Voltage":cluster{dbl[], dbl[]})  [unwired: 1 in]
              n603 = Bundle(w1801, w1827) -> (→"Current":cluster{dbl[], dbl[]})  [unwired: 1 in]
              n604 = Bundle(w1801, w1828) -> (→"Resistivity":cluster{dbl[], dbl[]})  [unwired: 1 in]
              n605 = Bundle(w1801, w1802) -> (→"Thermocouple (Sample holder 1) 2":cluster{dbl[], dbl[]})  [unwired: 1 in]
              n606 = Build Array (concatenate)(w1823, w1833, w1832, w1822, w1810, w1806, w1804) -> (w1840:dbl[])
              "appended array" <- w1840
            }
            frame #6 {
              n607 = Unbundle(w1849) -> ("COM out"=w1848:refnum<visa-resource-name>, "Cluster (Ausgang)"=w1847:errorcluster)
              n608 = Unbundle(w1846) -> ("COM out"=w1845:refnum<visa-resource-name>, "Cluster (Ausgang)"=w1844:errorcluster)
              n609 = case shown="True" "Write to File" {
                tunnel: [_ w1877] -> w1863
                tunnel: "File Path" -> [_ w1875]
                tunnel: w1856 -> [_ w1873]
                frame False {
                  n610 = property on="Write to File" class="Bool (strict)"("Blinking"=FALSE) -> ()  [unwired: 2 in, 2 out]
                }
                frame True {
                  n611 = flat-sequence {
                    tunnel: [w1879] -> w1876
                    tunnel: w1875 -> [w1879]
                    tunnel: [w1878] -> w1874
                    tunnel: w1873 -> [w1878]
                    tunnel: [w1884] -> w1877
                    tunnel: w1876 -> [w1883]
                    tunnel: w1874 -> [w1882]
                    frame #0 {
                      n612 = property on="Write to File" class="Bool (strict)"("Blinking"=TRUE) -> ()  [unwired: 2 in, 2 out]
                    }
                    frame #1 {
                      n613 = call-poly <vilib>:"Write To Spreadsheet File.vi"("format (%.3f)"="%g", "append to file? (new file:F)"=TRUE ("transpose? (no:F)"), "1D data"=w1882, "file path (dialog if empty)"=w1883) -> ("new file path (Not A Path if cancelled)"=w1884:path)  [unwired: 4 in]
                    }
                  }
                }
              }
              n614 = Merge Errors(w1868, w1867, w1865, w1847, w1844) -> (w1866:errorcluster)
              n615 = call <vilib>:"Simple Error Handler.vi"("error in (no error)"=w1866) -> ("error?"=w1850:bool)  [unwired: 4 in, 4 out]
              n616 = local write "File Path"(w1863) -> ()
            }
            frame #7 {
              w1903 = u32 1000 ("y")
              n617 = Tick Count (ms)() -> (millisecond timer value=w1905:u32)
              n618 = Subtract(x=w1905, y=w1904) -> (x-y=w1906:u32)
              n619 = VISA Flush I/O Buffer(VISA resource name=w1897, error in (no error)=w1896) -> (VISA resource name out=w1894:refnum<visa-resource-name>, error out=w1895:errorcluster)  [unwired: 1 in]
              n620 = VISA Flush I/O Buffer(VISA resource name=w1890, error in (no error)=w1889) -> (VISA resource name out=w1893:refnum<visa-resource-name>, error out=w1892:errorcluster)  [unwired: 1 in]
              n621 = Divide(x=w1906, y=w1903) -> (x/y=→"loop time (s)":dbl)
              n622 = Subtract(x="Intervall (s)", y=u32 1) -> (x-y=w1907:u32)
              n623 = Multiply(x=w1907, y=w1903) -> (x*y=w1910:u32)
              n624 = Wait (ms)(milliseconds to wait=w1910) -> ()  [unwired: 1 out]
              n625 = Bundle("COM out"=w1894, "error out"=w1895, "COM out"=w1893, "error out"=w1892) -> (w1891:T13)  [unwired: 1 in]
            }
            frame #8 {
              n626 = Tick Count (ms)() -> (millisecond timer value=w1933:u32)
              n627 = Subtract(x=w1933, y=w1931) -> (x-y=w1932:u32)
              n628 = Divide(x=w1932, y=w1930) -> (x/y=→"data logger intervall (s)":dbl)
            }
          }
          n629 = Exclusive Or(1:"stop", 2:w182) -> (0:w183:bool)
        }
      }
      frame #4 {
        n630 = call "VC840_Close.vi"("error in (no error)"=w1955, "VISA resource name"=w1956) -> ("error out"=w1964:errorcluster)  [unwired: 9 in]
        n631 = call "VC840_Close.vi"("error in (no error)"=w1957, "VISA resource name"=w1958) -> ("error out"=w1962:errorcluster)  [unwired: 9 in]
        n632 = VISA Close(VISA resource name=w1960, error in (no error)=w1959) -> (error out=w1961:errorcluster)
        n633 = VISA Close(VISA resource name=w1948, error in (no error)=w1947) -> (error out=w1946:errorcluster)
        n634 = Unbundle(w1953) -> ("COM out"=w1952:refnum<visa-resource-name>, "error out"=w1951:errorcluster, "COM out"=w1949:refnum<visa-resource-name>, "error out"=w1950:errorcluster)
        n635 = VISA Close(VISA resource name=w1952, error in (no error)=w1951) -> ()  [unwired: 1 out]
        n636 = VISA Close(VISA resource name=w1949, error in (no error)=w1950) -> ()  [unwired: 1 out]
        n637 = Merge Errors(w1961, w1962, w1964, w1946) -> (w1963:errorcluster)
        n638 = call <vilib>:"Simple Error Handler.vi"("error in (no error)"=w1963) -> ("error?"=w1954:bool)  [unwired: 1 in, 7 out]
        n639 = Stop(stop? (T)=w1954) -> ()
      }
    }
  }
